vi "engine-step-function.vi"(8 "error in (no error)":errorcluster, 9 "isRunning?":bool=TRUE, 10 "clk":dbl, 11 "HeaderElement in":cluster{variant[]}) -> (0 "error out":errorcluster, 1 "ENG.CALL":cluster{"CMD":T1, "data":variant}={"CMD"=enum."ENG.PROC.ISRUNNING", "data"=variant}, 2 "Next State in":cluster{"CMD":T2, "data":variant}={"CMD"=enum."JUMP", "data"=variant}, 3 "HeaderElement out":cluster{variant[]}, 4 "continue?":bool)   [LabVIEW 2024]
uses:
  controls/typeCmdPostStepFunc.ctl
  controls/state-engine.ctl
  controls/typeProcVarientName.ctl
  controls/type.StepFunction.ctl
  controls/enumVarCtrlIO.ctl
  controls/enum.io.mode.ctl
  controls/enum.io.type.ctl
  controls/IONode.ctl
  controls/type.address.ctl
  controls/typeXyPoint.ctl
  controls/typeStepVarients.ctl
  controls/typePathSelector.ctl
  controls/enum-q-sched.ctl
  controls/cluster-q-sched.ctl
  controls/type.eng.proc.isrunning.ctl
  controls/type.eng-call.proc-insert.ctl
  Polymorphics/variantCtrlStepFunction.vi
  Polymorphics/variantCtrlString.vi
  Polymorphics/variantCtrlSetpoint.vi
  Polymorphics/variantCtrlNumber.vi
  <vilib>/Utility/error.llb/Trim Whitespace.vi
  <vilib>/Utility/error.llb/Trim Whitespace One-Sided.vi
  Polymorphics/enumToStr.ProcHead.vi
  util.error.create.vi
  Polymorphics/variantCtrlStepPath.vi
  globals/globals-engine.vi
  util.environment.vi
  util-address-builder.vi
  util.DO.ToString.vi
  Polymorphics/io.command-builder.vi
  Polymorphics/io.command-builder.DO.vi
  Polymorphics/io.command-builder.AI.vi
  Polymorphics/io.command-builder.DI.vi
  io.frame.vi
  io.visa.vi
  io.responseValidator.vi
  Polymorphics/io.command-parser.DI.vi
  Polymorphics/io.command-parser.AI.vi
  <vilib>/Utility/libraryn.llb/Create Directory Recursive.vi
  Polymorphics/variantCtrlStepPointer.vi
  <vilib>/Utility/file.llb/Write Delimited Spreadsheet (string).vi
  Polymorphics/variantCtrlStepUserMessage.vi
  Polymorphics/variantCtrlStepProcPointer.vi
  Polymorphics/enumToStr.Step.vi
panel:
  out "DI":bool[](array[boolean])
  in  "deltaClk(global def)":dbl
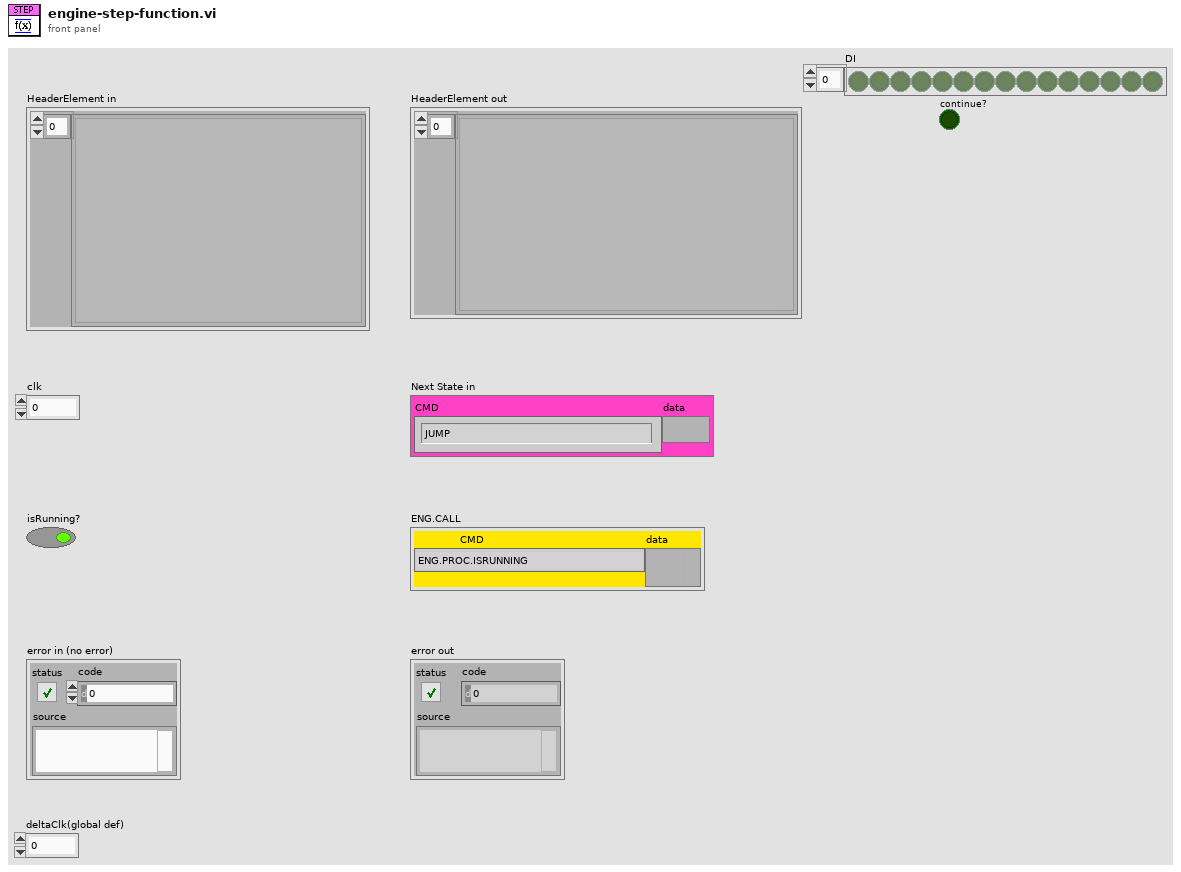
[diagram p1: front panel]
types:
  T1 = typedef "state-engine.ctl" = enum16{"ENG.NO-OP", "ENG.START", "ENG.STOP", "ENG.EXECUTE", "ENG.STATUS", "ENG.EXTERNAL-CALL", "ENG.INIT", "ENG.INIT.VARS", "ENG.INIT.SERIAL", "ENG.LOAD", "ENG.LOAD.SINGLE", "ENG.LOAD.MODULE", "ENG.LOAD.RELOAD", "ENG.LOAD.UNLOAD", "ENG.IO.LOAD", "ENG.IO.SAVE", "ENG.PROC.RELOAD-BY-NAME", "ENG.PROC.START", "ENG.PROC.STOP", "ENG.PROC.INSERT-STEPS", "ENG.PROC.ISRUNNING", "ENG.PROC.PRESET", "ENG.PROC.STATUS", "ENG.PRINT-USER-MSG", "ENG.RIO.SNAPSHOT", "ENG.RIO.AIN-SNAPSHOT-CALIB", "ENG.RIO.DOUT-BY-ADDR", "ENG.RIO.DOUT-BY-NAME", "ENG.RIO.RFS-DELAY-SET-X1", "ENG.RIO.RFS-DELAY-SET-X8", "ENG.RIO.RFS-CYCLES-SET", "ENG.RIO.RFS-CYCLES-GET", "ENG.RIO.RFS-ENABLE", "ENG.EXIT"}
  T2 = typedef "typeCmdPostStepFunc.ctl" = enum16{"NEXT", "PREV", "JUMP", "STAY", "COMPLETE", "ENGCALL.PROC.START", "ENGCALL.PROC.STOP", "ENGCALL.PROC.COMPLETION-CHECK", "ENGCALL.PROC.INIT", "ERROR"}
  T3 = typedef "typeProcVarientName.ctl" = enum16{"procNameID", "procModuleID", "procPath", "procIsRunning", "procIndex", "procModule", "procRegisterNumeric", "procRegisterString", "procReport", "procReportPrev", "procCLK", "procStepPointer", "procType"}
  T4 = typedef "enumVarCtrlIO.ctl" = enum16{"IO Get By Key", "IO List Configs", "IO Add By Key", "IO Modify Value By Key", "IO Modify Calib By Key", "IO Modify ADDR By Key", "IO Modify Mode By Key", "IO Modify Type By Key", "IO Modify Name By Key", "IO Remove By Key", "IO Remove All"}
  T5 = typedef "IONode.ctl" = cluster{"ADDR":T6, "Label":string, "Type":T7, "Mode":T8, "Value":string, "Tags":string, "calibration":T9[]}
  T6 = typedef "type.address.ctl" = u16
  T7 = typedef "enum.io.type.ctl" = enum16{"Type", "DI", "DO", "AI", "AO", "VL", "BUF"}
  T8 = typedef "enum.io.mode.ctl" = enum16{"Mode", "RIO", "SIM"}
  T9 = typedef "typeXyPoint.ctl" = cluster{"X":dbl, "Y":dbl}
  T10 = typedef "typeStepVarients.ctl" = enum16{"stepNameID", "stepFunction", "stepReport", "stepSetpoint", "stepPointer", "stepProcPointer", "stepIoPointer", "stepIoValue", "stepFilePointer", "stepMessage", "stepTimeString", "stepNumReg", "stepStrReg", "stepSeconds", "stepUnitDoseParams", "stepUnitIndex"}
  T11 = typedef "typePathSelector.ctl" = enum16{"DIR_PROCS", "DIR_CONFIG", "DIR_TEMPLATE", "DIR_IO_FILE", "DIR_RECORD", "DIR_LOG", "DIR_RUNTIME", "DIR_PRESET", "DIR_INI"}
  T12 = typedef "cluster-q-sched.ctl" = cluster{"Proc Name":string, "value":cluster{"Enable":bool, "Time":timestamp}}
  T13 = typedef "enum-q-sched.ctl" = enum16{"SCHED.INIT", "SCHED.REGISTER", "SCHED.EXIT"}
  T14 = typedef "type.eng.proc.isrunning.ctl" = cluster{"callerProc":string, "procPointer":string}
  T15 = typedef "type.eng-call.proc-insert.ctl" = cluster{"ProcName":string, "instructions":variant[]}
  T16 = typedef "type.StepFunction.ctl" = enum16{"__NO-OP", "_DELAY_LOAD", "_DELAY_COMPARE", "_JUMP", "_COMPLETE", "_COMPARE", "_LOG_MESSAGE", "_LOG_LAST_REPORT", "_SCHEDULE", "_SCHEDULE_DAILY", "CLK_COMPARE", "PROC_START", "PROC_STOP", "PROC_LOAD", "PROC_COMPLETION_CHECK", "PROC_COMPLETION_LOAD", "_IO_READ", "_IO_READ_MANY", "_IO_WRITE", "_IO_WRITE_BY_REG", "_IO_GET_OUTPUT", "_OCS_CHECK", "_OCS_RECORD", "_GET_RH", "_GET_ACC_UV", "_GET_WD", "_GET_WS", "_REC_DELETE", "_REC_MOVE", "_REC_COPY", "_IRR_CHECK", "UNIT_CHECK", "UNIT_SAMPLE", "UNIT_DOSE"}
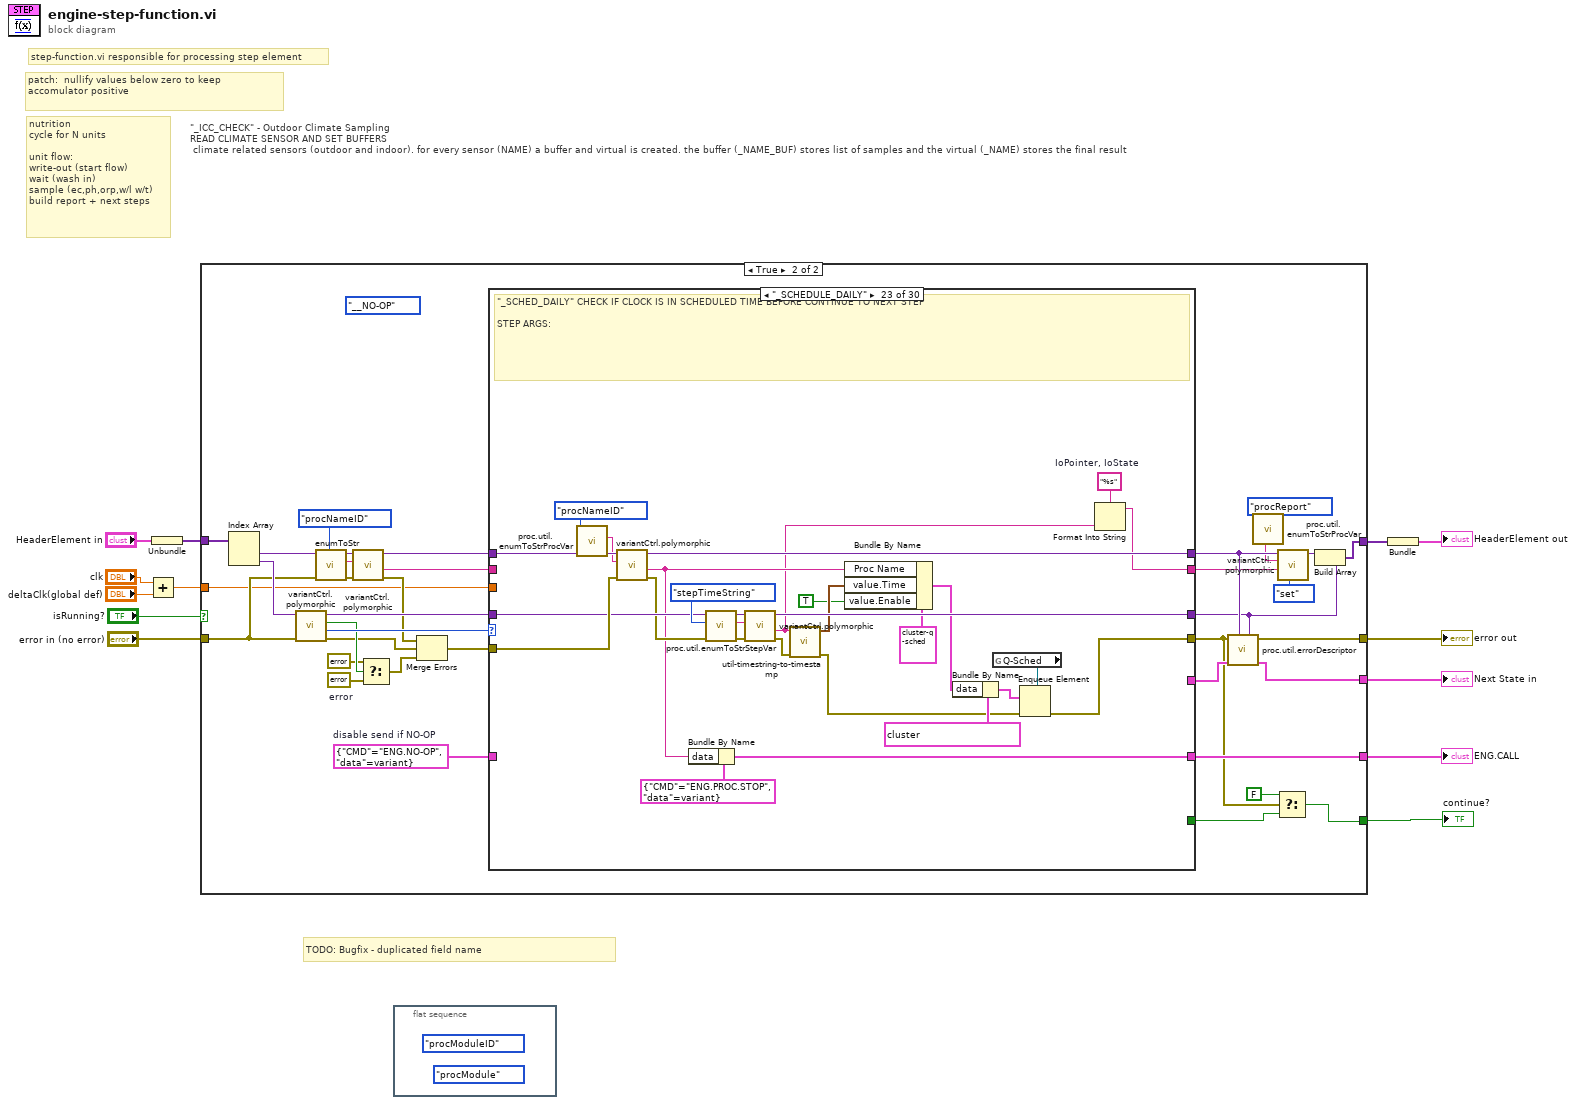
[diagram p0: block diagram]
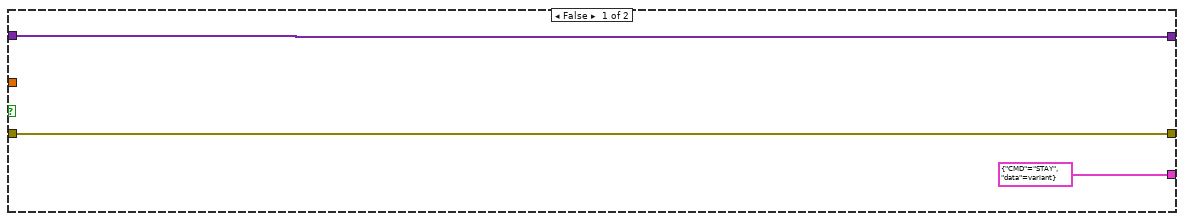
[diagram p2: hidden frame]
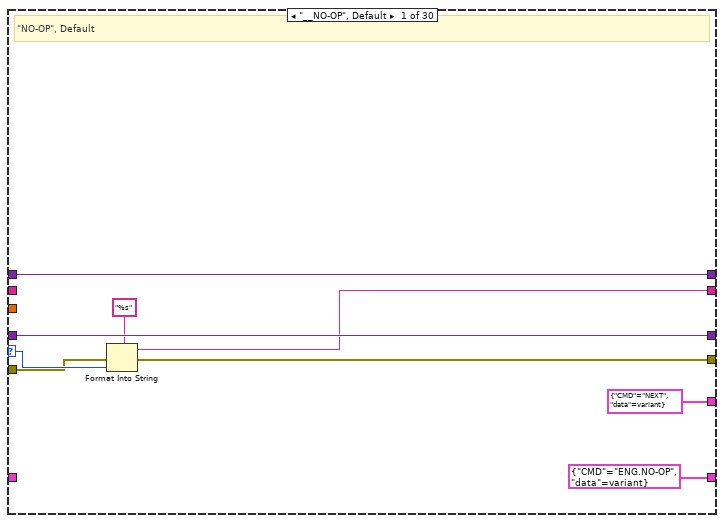
[diagram p3: hidden frame]
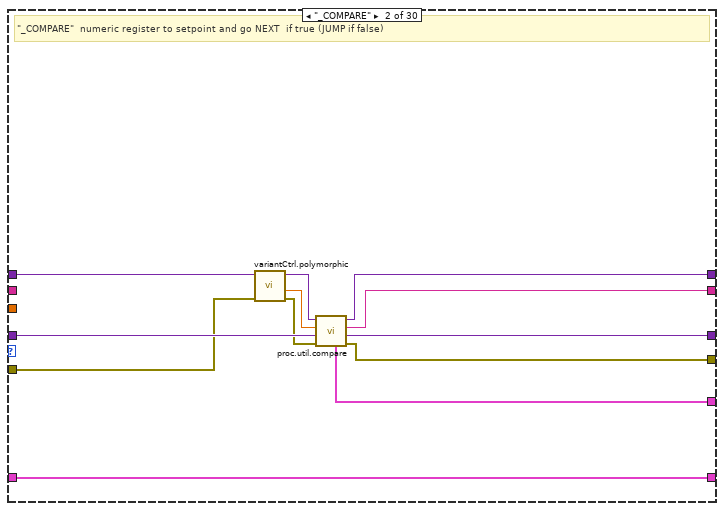
[diagram p4: hidden frame]
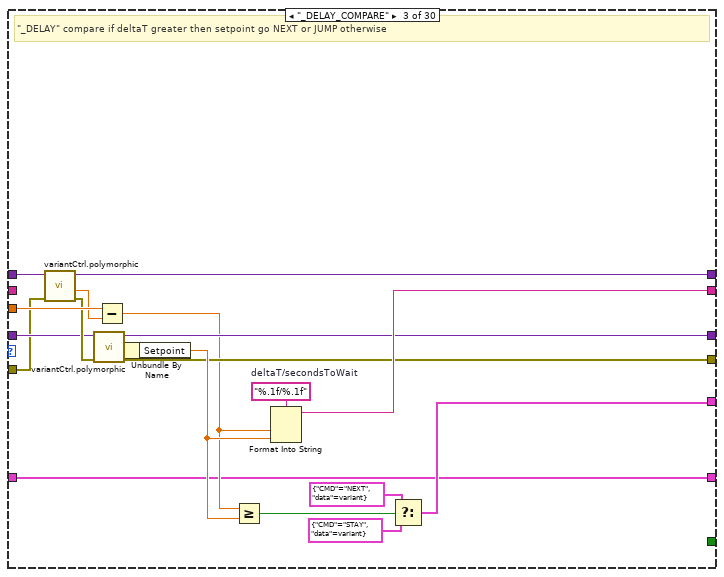
[diagram p5: hidden frame]
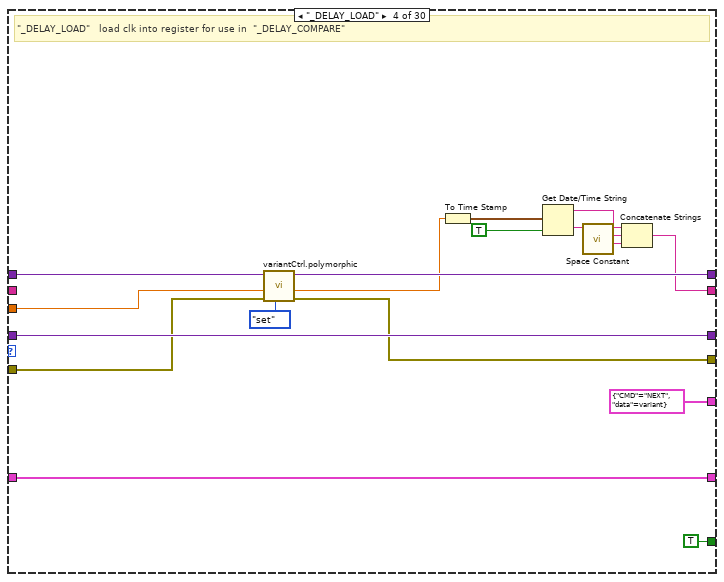
[diagram p6: hidden frame]
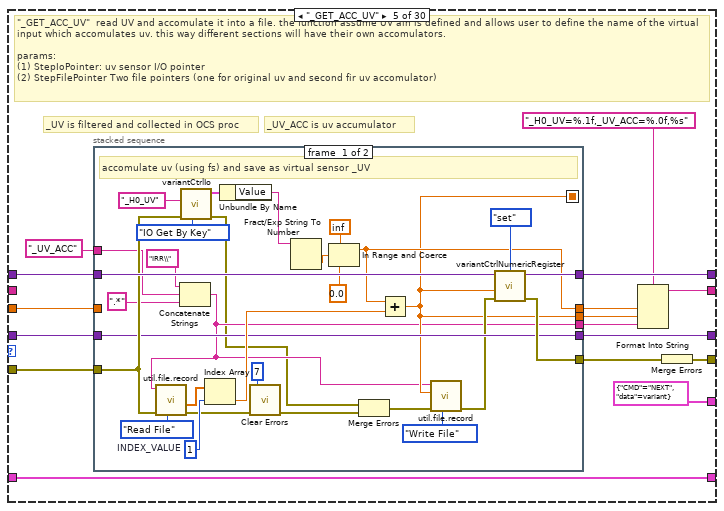
[diagram p7: hidden frame]
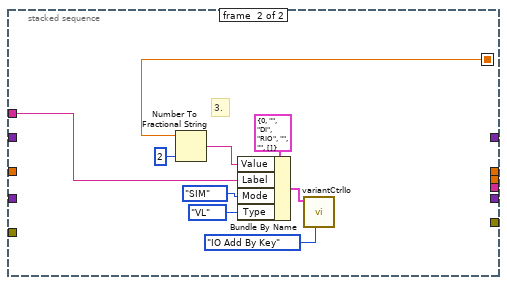
[diagram p8: hidden frame]
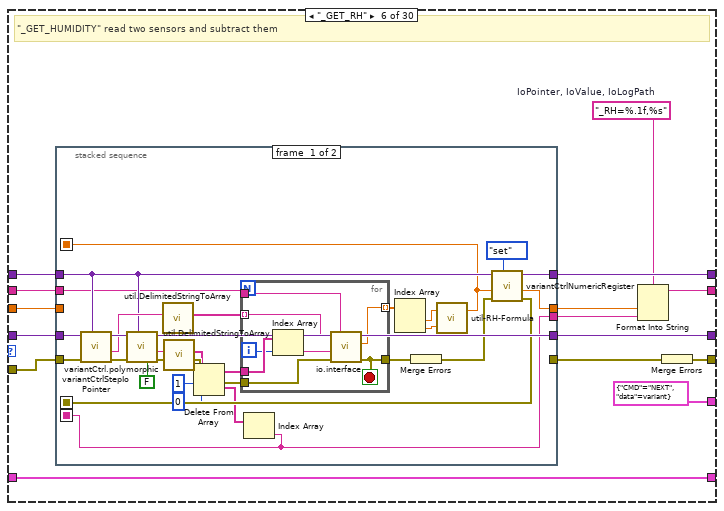
[diagram p9: hidden frame]
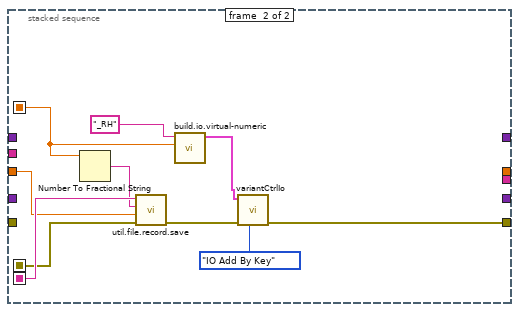
[diagram p10: hidden frame]
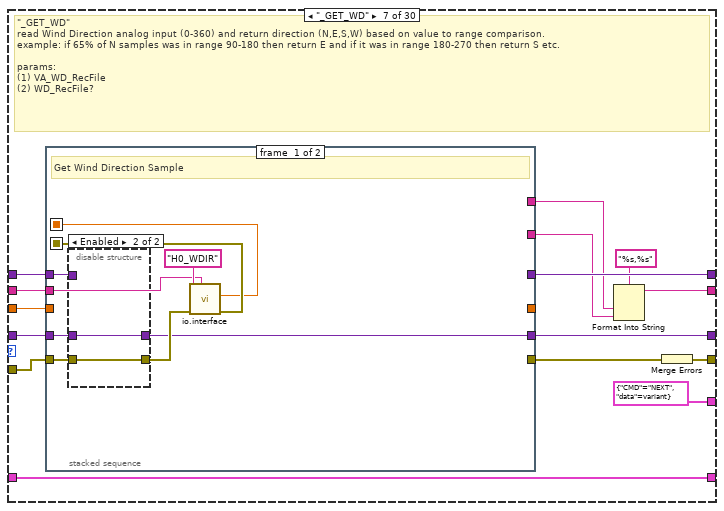
[diagram p11: hidden frame]
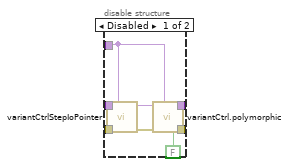
[diagram p12: hidden frame]
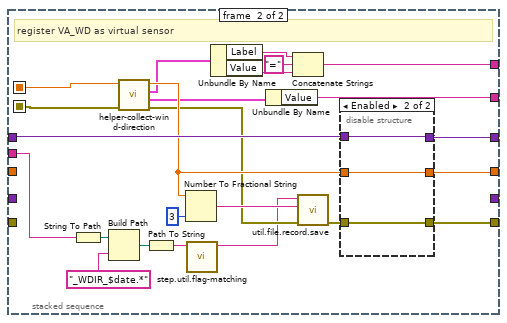
[diagram p13: hidden frame]
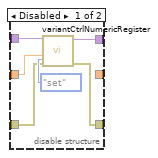
[diagram p14: hidden frame]
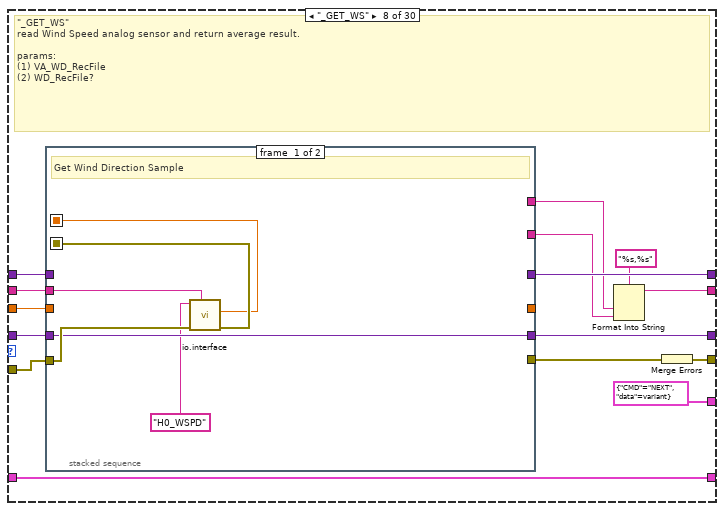
[diagram p15: hidden frame]
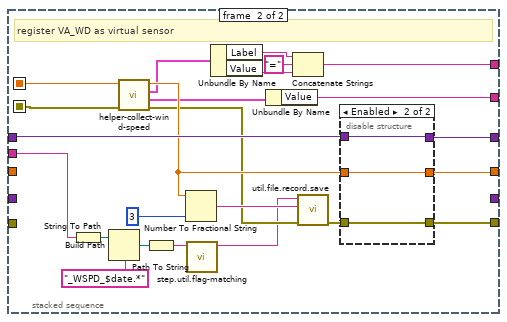
[diagram p16: hidden frame]
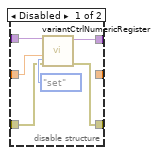
[diagram p17: hidden frame]
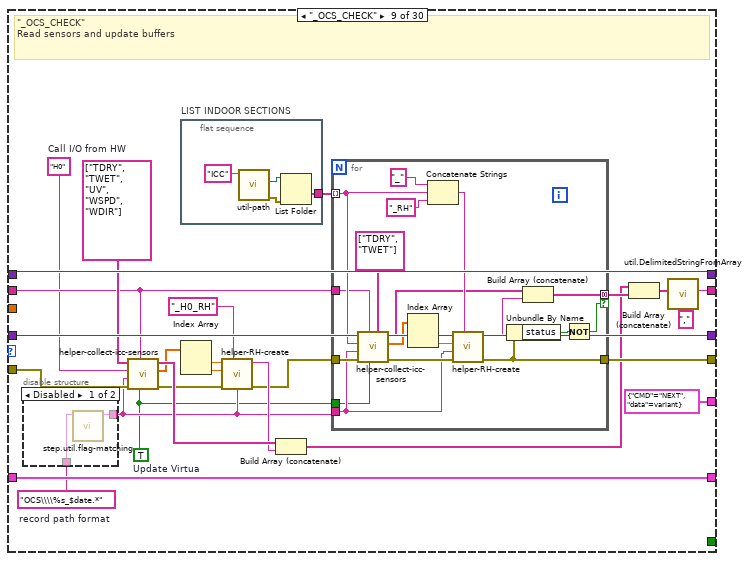
[diagram p18: hidden frame]
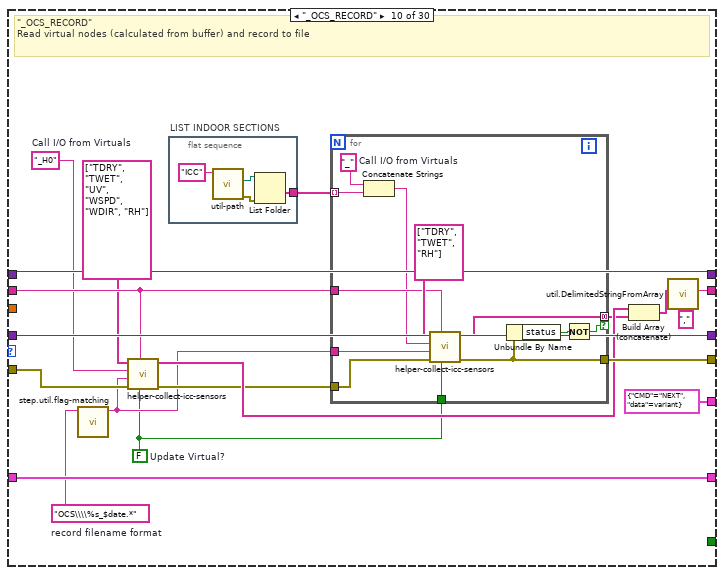
[diagram p20: hidden frame]
diagram:
  # "TODO: Bugfix - duplicated field name"
  # "\"_ICC_CHECK\" - Outdoor Climate Sampling\nREAD CLIMATE SENSOR AND SET BUFFERS\n climate related sensors (outdoor and indoor). for every sensor (NAME) a buffer and virtual is created. the buffer (_NAME_BUF) stores list of samples and the virtual (_NAME) stores the final result"
  # "patch:  nullify values below zero to keep accomulator positive"
  # "nutrition\ncycle for N units\n\nunit flow:\nwrite-out (start flow)\nwait (wash in)\nsample (ec,ph,orp,w/l w/t)\nbuild report + next steps"
  # "step-function.vi responsible for processing step element"
  n1 = Add(x="clk", y="deltaClk(global def)") -> (x+y=w2:dbl)
  n2 = Unbundle("HeaderElement in") -> (w7:variant[])
  n3 = case shown="True" "isRunning?" {
    tunnel: [cluster{"CMD":T2, "data":variant} {"CMD"=enum."STAY", "data"=variant} ("Next State") w33] -> w13
    tunnel: [w15 w32] -> w12
    tunnel: [w16 w46] -> w11
    tunnel: w7 -> [w16 w39]
    tunnel: "error in (no error)" -> [w15 w37]
    tunnel: w2 -> [_ w35]
    tunnel: [_ w27] -> w5
    tunnel: [_ w17] -> w1
    frame False {
    }
    frame True {
      w26 = cluster{"CMD":T1, "data":variant} {"CMD"=enum."ENG.NO-OP", "data"=variant}  # disable send if NO-OP
      (unwired) type.StepFunction."__NO-OP" ("Operation out")
      w44 = errorcluster {"status"=TRUE, "code"=-1, "source"="Missing stepFunction "}  # error
      n4 = Index Array(array=w39) -> (element #1=w40:variant, element #2=w38:variant)  [unwired: 2 in]
      n5 = call-poly "variantCtrl.polymorphic.vi"("error in"=w37, "variant in"=w38) -> ("error out"=w41:errorcluster, "StepFunction"=w50:T16, "found/replaced"=w45:bool, "variant out"=w51:variant)  [unwired: 6 in]
      n6 = call-poly "enumToStr.vi"("Proc var"=typeProcVarientName."procNameID" ("proc var")) -> ("String"=w21:string)  [unwired: 10 in]
      n7 = call-poly "variantCtrl.polymorphic.vi"("error in"=w37, "name in"=w21, "Step in"=w40) -> ("error out"=w36:errorcluster, "String Value"=w24:string, "Step out"=w49:variant)  [unwired: 5 in, 1 out]
      n8 = Select(t=errorcluster {"status"=FALSE, "code"=0, "source"=""}, s=w45, f=w44) -> (s? t:f=w43:errorcluster)
      n9 = Merge Errors(w36, w41, w43) -> (w48:errorcluster)
      n10 = case "Step Functions" shown="\"_SCHEDULE_DAILY\"" w50 {
        selector: w50 -> [w57 _ _ _ _ _ _ _ _ _ _ _ _ _ _ _ _ _ _ _ w728 _ _ _ _ _ w864 _ _ _]
        tunnel: w51 -> [w59 w67 w82 w108 w121 w175 w236 w303 w370 w414 w446 w493 w524 w554 w576 w587 w613 w621 w650 w663 w746 w769 w787 w802 w826 w860 w870 w892 w911 w968]
        tunnel: [w53 w66 w80 w105 w116 w170 w231 w298 w363 w410 w442 w489 w519 w549 w574 w580 w608 w616 w644 w661 w741 w768 w785 w800 w817 w838 w868 w881 w906 w958] -> w20
        tunnel: [w59 w69 w81 w108 w122 w176 w237 w304 w370 w414 w447 w494 w523 w551 w575 w588 w612 w621 w651 w658 w747 w771 w788 w805 w825 w859 w869 w893 w912 w969] -> w30
        tunnel: w35 -> [_ _ w91 w100 w114 w168 w229 w296 _ _ _ _ _ _ _ w594 _ _ _ _ _ w764 _ w803 _ _ _ w879 _ _]
        tunnel: w49 -> [w60 w71 w87 w107 w120 w174 w235 w302 w369 w413 w444 w491 w522 w545 w568 w595 w611 w618 w649 w659 w745 w763 w794 w806 w821 w853 w862 w896 w914 w972]
        tunnel: [w60 w72 w83 w106 w123 w177 w238 w305 w369 w413 w448 w495 w522 w545 w569 w595 w611 w619 w654 w665 w745 w763 w795 w807 w822 w840 w862 w896 w914 w972] -> w31
        tunnel: [w55 w64 w88 w94 w117 w171 w232 w299 w366 w411 w450 w498 w512 w558 w577 w593 w606 "completed" ("status") w639 w660 w742 w767 w774 w799 w813 w851 w861 w884 w904 w957] -> w22
        tunnel: [cluster{"CMD":T2, "data":variant} {"CMD"=enum."NEXT", "data"=variant} ("Next State") w68 w77 cluster{"CMD":T2, "data":variant} {"CMD"=enum."NEXT", "data"=variant} ("Next State") cluster{"CMD":T2, "data":variant} {"CMD"=enum."NEXT", "data"=variant} ("Next State") cluster{"CMD":T2, "data":variant} {"CMD"=enum."NEXT", "data"=variant} ("Next State") cluster{"CMD":T2, "data":variant} {"CMD"=enum."NEXT", "data"=variant} ("Next State") cluster{"CMD":T2, "data":variant} {"CMD"=enum."NEXT", "data"=variant} ("Next State") cluster{"CMD":T2, "data":variant} {"CMD"=enum."NEXT", "data"=variant} ("Next State") cluster{"CMD":T2, "data":variant} {"CMD"=enum."NEXT", "data"=variant} ("Next State") cluster{"CMD":T2, "data":variant} {"CMD"=enum."NEXT", "data"=variant} ("Next State") cluster{"CMD":T2, "data":variant} {"CMD"=enum."NEXT", "data"=variant} ("Next State") cluster{"CMD":T2, "data":variant} {"CMD"=enum."NEXT", "data"=variant} ("Next State") cluster{"CMD":T2, "data":variant} {"CMD"=enum."NEXT", "data"=variant} ("Next State") cluster{"CMD":T2, "data":variant} {"CMD"=enum."NEXT", "data"=variant} ("Next State") w583 w609 cluster{"CMD":T2, "data":variant} {"CMD"=enum."COMPLETE", "data"=variant} ("JUMP") cluster{"CMD":T2, "data":variant} {"CMD"=enum."NEXT", "data"=variant} ("JUMP") w664 cluster{"CMD":T2, "data":variant} {"CMD"=enum."NEXT", "data"=variant} ("Next State") w770 _ w804 w819 cluster{"CMD":T2, "data":variant} {"CMD"=enum."NEXT", "data"=variant} ("Next State") cluster{"CMD":T2, "data":variant} {"CMD"=enum."NEXT", "data"=variant} ("Next State") cluster{"CMD":T2, "data":variant} {"CMD"=enum."NEXT", "data"=variant} ("Next State") w913 cluster{"CMD":T2, "data":variant} {"CMD"=enum."NEXT", "data"=variant} ("Next State")] -> w34
        tunnel: w48 -> [w54 w62 w75 w102 w119 w173 w234 w301 w355 w409 w441 w487 w521 w543 w572 w582 w605 w617 w648 w662 w744 w766 w791 w801 w815 w850 w867 w882 _ _]
        tunnel: [cluster{"CMD":T1, "data":variant} {"CMD"=enum."ENG.NO-OP", "data"=variant} ("element") w61 w73 w101 w110 w165 w228 w295 w368 w412 w440 w484 w520 w541 w570 w591 w604 w620 w628 w657 w726 w765 w796 w798 w809 w848 w865 w889 w909 w963] -> w27
        tunnel: w26 -> [_ w61 w73 w101 w110 w165 w228 w295 w368 w412 w440 w484 w520 w541 w570 w590 w604 w620 w628 w657 w726 w765 _ w798 w809 _ _ w891 w910 w965]
        tunnel: w24 -> [_ _ _ _ _ w164 w227 w294 w351 w408 w432 w480 w510 w538 w561 w589 _ _ _ _ _ _ _ _ _ _ _ w887 w908 w956]
        tunnel: [_ _ _ TRUE _ _ _ _ _ _ _ _ _ TRUE _ _ _ _ _ _ _ _ _ _ _ _ _ _ _ _] -> w18
        frame "__NO-OP", Default {
          # "\"NO-OP\", Default"
          n11 = Format Into String(format string="%s", error in=w54, w57) -> (resulting string=w55:string, error out=w53:errorcluster)  [unwired: 1 in]
        }
        frame "_COMPARE" {
          # "\"_COMPARE\"  numeric register to setpoint and go NEXT  if true (JUMP if false)"
          n12 = call-poly "variantCtrl.polymorphic.vi"("error in"=w62, "procElement"=w71) -> ("error out"=w63:errorcluster, "procNumericRegister out"=w65:dbl, "procElement out"=w70:variant)  [unwired: 7 in]
          n13 = call "proc.util.compare.vi"("error in"=w63, "stepElement in"=w67, "Input"=w65, "procElement in"=w70) -> ("error out"=w66:errorcluster, "stepElement out"=w69:variant, "resulting string"=w64:string, "procElement out"=w72:variant, "Next State"=w68:cluster{"CMD":T2, "data":variant})  [unwired: 3 in]
        }
        frame "_DELAY_COMPARE" {
          w90 = "%.1f/%.1f"  # deltaT/secondsToWait
          # "\"_DELAY\" compare if deltaT greater then setpoint go NEXT or JUMP otherwise"
          n14 = call-poly "variantCtrl.polymorphic.vi"("error in"=w75, "procElement"=w87) -> ("error out"=w86:errorcluster, "procNumericRegister out"=w85:dbl, "procElement out"=w83:variant)  [unwired: 7 in]
          n15 = call-poly "variantCtrl.polymorphic.vi"("error in"=w86, "procElement in in"=w82) -> ("error out"=w80:errorcluster, "setpoint"=w89:cluster{"Comparison":string, "Setpoint":dbl}, "procElement out"=w81:variant)  [unwired: 6 in, 1 out]
          n16 = Subtract(x=w91, y=w85) -> (x-y=w79:dbl)
          n17 = Unbundle By Name(w89) -> ("Setpoint"=w84:dbl)
          n18 = Greater Or Equal?(x=w79, y=w84) -> (x >= y?=w78:bool)
          n19 = Format Into String(format string=w90, w79, w84) -> (resulting string=w88:string)  [unwired: 2 in, 1 out]
          n20 = Select(t=cluster{"CMD":T2, "data":variant} {"CMD"=enum."NEXT", "data"=variant} ("NEXT"), s=w78, f=cluster{"CMD":T2, "data":variant} {"CMD"=enum."STAY", "data"=variant} ("JUMP")) -> (s? t:f=w77:cluster{"CMD":T2, "data":variant})
        }
        frame "_DELAY_LOAD" {
          # "\"_DELAY_LOAD\"   load clk into register for use in  \"_DELAY_COMPARE\""
          n21 = call-poly "variantCtrl.polymorphic.vi"("menu"=enum16{"get", "set"}."set", "error in"=w102, "procNumericRegister in"=w100, "procElement"=w107) -> ("error out"=w105:errorcluster, "procNumericRegister out"=w99:dbl, "procElement out"=w106:variant)  [unwired: 5 in]
          n22 = To Time Stamp(1:w99) -> (0:w98:timestamp)
          n23 = Get Date/Time String(seconds (now)=w98, want seconds? (F)=TRUE) -> (date string=w95:string, time string=w97:string)  [unwired: 1 in]
          n24 = call <vilib>:"Space Constant.vi"() -> ("String"=w96:string)
          n25 = Concatenate Strings(w97, w96, w95) -> (w94:string)
        }
        frame "_GET_ACC_UV" {
          # "_UV_ACC is uv accumulator"
          # "_UV is filtered and collected in OCS proc"
          # "\"_GET_ACC_UV\"  read UV and accomulate it into a file. the function assume UV ain is defined and allows user to define the name of the virtual input which accomulates uv. this way different sections will have their own accomulators. \n\nparams:\n(1) StepIoPointer: uv sensor I/O pointer\n(2) StepFilePointer Two file pointers (one for original uv and second fir uv accomulator)"
          n26 = stacked-sequence {
            seq-local: [w130 _] -> [_ w158]
            tunnel: [w154 _] -> w123
            tunnel: [w137 _] -> w122
            tunnel: w121 -> [w137 _]
            tunnel: w120 -> [w152 _]
            tunnel: w119 -> [w138 _]
            tunnel: [w153 _] -> w115
            tunnel: w114 -> [_ _]
            tunnel: [w132 _] -> w113
            tunnel: [w127 _] -> w112
            tunnel: [w130 _] -> w111
            tunnel: "_UV_ACC" ("Label") -> [w129 w155]
            frame #0 {
              w149 = 1  # INDEX_VALUE
              # "accomulate uv (using fs) and save as virtual sensor _UV"
              n27 = Concatenate Strings("IRR\\" ("string"), w129, ".*" ("$string in")) -> (w127:string)
              n28 = call "util.file.record.vi"("Operation(Read)"=enum16{"Read File", "Write File"}."Read File", "error in"=w138, "path.* in"=w127) -> ("error out"=w147:errorcluster, "Last Record out"=w150:dbl[])  [unwired: 5 in, 2 out]
              n29 = call "variantCtrlIo.vi"("menu (Get Param)"=enumVarCtrlIO."IO Get By Key", "error in"=w138, "Key (use IOnode Label if empty )"="_H0_UV" ("Label")) -> ("error out"=w126:errorcluster, "IOnode out"=w140:T5)  [unwired: 4 in, 3 out]
              n30 = Index Array(array=w150, index=w149) -> (element=w148:dbl)
              n31 = Unbundle By Name(w140) -> ("Value"=w139:string)
              n32 = call <vilib>:"Clear Errors.vi"("error in (no error)"=w147, "specific error code to clear (0: all)"=7) -> ("error out"=w145:errorcluster)  [unwired: 4 in, 1 out]
              n33 = Fract/Exp String To Number(string=w139) -> (number=w135:dbl)  [unwired: 3 in, 1 out]
              n34 = In Range and Coerce(upper limit=inf, x=w135, lower limit=0.0) -> (coerced(x)=w132:dbl)  [unwired: 1 out]
              n35 = Merge Errors(w126, w145) -> (w136:errorcluster)
              n36 = Add(x=w132, y=w148) -> (x+y=w130:dbl)
              n37 = call "util.file.record.vi"("Operation(Read)"=enum16{"Read File", "Write File"}."Write File", "error in"=w136, "value"=w130, "path.* in"=w127) -> ("error out"=w131:errorcluster)  [unwired: 4 in, 3 out]
              n38 = call "variantCtrlNumericRegister.vi"("menu"=enum16{"get", "set"}."set", "error in"=w131, "procNumericRegister in"=w130, "procElement"=w152) -> ("error out"=w153:errorcluster, "procElement out"=w154:variant)  [unwired: 5 in, 1 out]
            }
            frame #1 {
              # "3."
              n39 = Number To Fractional String(number=w158, precision (6)=i16 2) -> (F-format string=w157:string)  [unwired: 2 in]
              n40 = Bundle By Name(cluster=T5 {"ADDR"=0, "Label"="", "Type"=enum."DI", "Mode"=enum."RIO", "Value"="", "Tags"="", "calibration"=[]} ("IoConf in"), "Value"=w157, "Label"=w155, "Mode"=enum.io.mode."SIM", "Type"=enum.io.type."VL" ("type")) -> (w161:T5)
              n41 = call "variantCtrlIo.vi"("menu (Get Param)"=enumVarCtrlIO."IO Add By Key" ("menu in (get)"), "IOnode in"=w161) -> ()  [unwired: 5 in, 5 out]
            }
          }
          n42 = Format Into String(format string="_H0_UV=%.1f,_UV_ACC=%.0f,%s", w113, w111, w112) -> (resulting string=w117:string)  [unwired: 2 in, 1 out]
          n43 = Merge Errors(w115) -> (w116:errorcluster)
        }
        frame "_GET_RH" {
          w172 = "_RH=%.1f,%s"  # IoPointer, IoValue, IoLogPath
          # "\"_GET_HUMIDITY\" read two sensors and subtract them"
          n44 = stacked-sequence {
            seq-local: [w180 _] -> [_ w216]
            seq-local: [w190 _] -> [_ w221]
            seq-local: [w186 _] -> [_ w222]
            tunnel: [w195 _] -> w177
            tunnel: [w194 _] -> w176
            tunnel: w175 -> [w204 _]
            tunnel: w174 -> [w193 _]
            tunnel: w173 -> [w202 _]
            tunnel: [_ w224] -> w169
            tunnel: w168 -> [_ w220]
            tunnel: [w189 _] -> w167
            tunnel: [w186 _] -> w166
            tunnel: w164 -> [w179 _]
            frame #0 {
              n45 = call "variantCtrlStepIoPointer.vi"("procElement"=w193, "error in"=w202, "StepElement in"=w204) -> ("error out"=w205:errorcluster, "I/O Pointer out"=w198:string, "stepElement out"=w203:variant)  [unwired: 5 in, 1 out]
              n46 = call-poly "variantCtrl.polymorphic.vi"("isRequired (T)"=FALSE, "procElement"=w193, "error in (no error)"=w205, "stepElement in"=w203) -> ("error out"=w206:errorcluster, "File Pointer out"=w196:string, "step\\element out"=w194:variant)  [unwired: 5 in]
              n47 = call "util.DelimitedStringToArray.vi"("delimitaed string"=w198) -> ("array out"=w197:string[])  [unwired: 10 in]
              n48 = call "util.DelimitedStringToArray.vi"("delimitaed string"=w196) -> ("array out"=w192:string[])  [unwired: 10 in]
              n49 = Delete From Array(array=w192, length=1, index=0) -> (deleted portion=w185:string[], array with subset deleted=w184:string[])
              n50 = for {
                tunnel: [w212] -> w199 mode=indexing
                tunnel: w197 -> [w213] mode=indexing
                tunnel: w184 -> [w210]
                tunnel: w206 -> [w214]
                tunnel: [w211] -> w200
                tunnel: w179 -> [w207]
                i -> [w209]
                stop <- w211 stop-if-true
                n51 = Index Array(array=w210, index=w209) -> (element=w208:string)
                n52 = call "io.interface.vi"("Caller"=w207, "error in"=w214, "record filename.* (disabled if empty)"=w208, "IO Name in"=w213) -> ("error out"=w211:errorcluster, "Value out"=w212:dbl)  [unwired: 2 in, 4 out]
              }
              n53 = Index Array(array=w185) -> (element=w186:string)  [unwired: 1 in]
              n54 = Index Array(array=w199) -> (element #1=w182:dbl, element #2=w181:dbl)  [unwired: 2 in]
              n55 = Merge Errors(w200) -> (w191:errorcluster)
              n56 = call "util-RH-Formula.vi"("Twet"=w181, "Tdry"=w182) -> ("RH"=w180:dbl)  [unwired: 1 out]
              n57 = call "variantCtrlNumericRegister.vi"("menu"=enum16{"get", "set"}."set", "error in"=w191, "procNumericRegister in"=w180, "procElement"=w193) -> ("error out"=w190:errorcluster, "procNumericRegister out"=w189:dbl, "procElement out"=w195:variant)  [unwired: 5 in]
            }
            frame #1 {
              n58 = Number To Fractional String(number=w216) -> (F-format string=w219:string)  [unwired: 3 in]
              n59 = call "util.file.record.save.vi"("error in"=w221, "clk(NaN)"=w220, "String Delimited Values"=w219, "record path in"=w222) -> ("error out"=w218:errorcluster)  [unwired: 6 in, 1 out]
              n60 = call "build.io.virtual-numeric.vi"("Numeric Value"=w216, "Label"="_RH" ("Virtual _RH")) -> ("IoConf out"=w215:T5)  [unwired: 9 in]
              n61 = call "variantCtrlIo.vi"("menu (Get Param)"=enumVarCtrlIO."IO Add By Key" ("menu in (get)"), "error in"=w218, "IOnode in"=w215) -> ("error out"=w224:errorcluster)  [unwired: 4 in, 4 out]
            }
          }
          n62 = Format Into String(format string=w172, w167, w166) -> (resulting string=w171:string)  [unwired: 2 in, 1 out]
          n63 = Merge Errors(w169) -> (w170:errorcluster)
        }
        frame "_GET_WD" {
          # "\"_GET_WD\" \nread Wind Direction analog input (0-360) and return direction (N,E,S,W) based on value to range comparison. \nexample: if 65% of N samples was in range 90-180 then return E and if it was in range 180-270 then return S etc. \n\nparams:\n(1) VA_WD_RecFile\n(2) WD_RecFile?"
          n64 = stacked-sequence {
            seq-local: [w242 _] -> [_ w279]
            seq-local: [w243 _] -> [_ w266]
            tunnel: [_ w282] -> w238
            tunnel: [w245 _] -> w237
            tunnel: w236 -> [w247 _]
            tunnel: w235 -> [w244 w280]
            tunnel: w234 -> [w246 _]
            tunnel: [_ w281] -> w230
            tunnel: w229 -> [_ _]
            tunnel: [_ w278] -> _
            tunnel: w227 -> [w240 w272]
            tunnel: [_ w264] -> w225
            tunnel: [_ w259] -> w226
            frame #0 {
              # "Get Wind Direction Sample"
              n65 = disable-structure shown="Enabled" {
                disable-tunnel: [w256 w257] -> w248
                disable-tunnel: w247 -> [w254 w258]
                disable-tunnel: w246 -> [w252 w257]
                disable-tunnel: [w250 w258] -> w245
                disable-tunnel: w244 -> [w249 _]
                frame Disabled {
                  n66 = call "variantCtrlStepIoPointer.vi"("procElement"=w249, "error in"=w252, "StepElement in"=w254) -> ("error out"=w255:errorcluster, "stepElement out"=w253:variant)  [unwired: 5 in, 2 out]
                  n67 = call-poly "variantCtrl.polymorphic.vi"("isRequired (T)"=FALSE, "procElement"=w249, "error in (no error)"=w255, "stepElement in"=w253) -> ("error out"=w256:errorcluster, "step\\element out"=w250:variant)  [unwired: 5 in, 1 out]
                }
                frame Enabled {
                }
              }
              n68 = call "io.interface.vi"("Caller"=w240, "error in"=w248, "IO Name in"="H0_WDIR") -> ("error out"=w243:errorcluster, "Value out"=w242:dbl)  [unwired: 3 in, 4 out]
            }
            frame #1 {
              # "register VA_WD as virtual sensor"
              n69 = String To Path(string=w272) -> (path=w271:path)
              n70 = Build Path(base path=w271, name or relative path="_WDIR_$date.*" ("record path in")) -> (appended path=w269:path)
              n71 = call "helper-collect-wind-direction.vi"("error in"=w266, "Value in"=w279) -> ("error out"=w274:errorcluster, "BUF Node"=w265:T5, "Result Node"=w263:T5, "Result"=w276:dbl)  [unwired: 6 in]
              n72 = Path To String(path=w269) -> (string=w268:string)
              n73 = Number To Fractional String(number=w276, precision (6)=i16 3) -> (F-format string=w275:string)  [unwired: 2 in]
              n74 = call "step.util.flag-matching.vi"("$string in"=w268) -> ("formated string out"=w267:string)  [unwired: 10 in]
              n75 = Unbundle By Name(w263) -> ("Label"=w262:string, "Value"=w261:string)
              n76 = Unbundle By Name(w265) -> ("Value"=w264:string)
              n77 = Concatenate Strings(w262, "=" ("string"), w261) -> (w259:string)
              n78 = call "util.file.record.save.vi"("error in"=w274, "String Delimited Values"=w275, "record path in"=w267) -> ("error out"=w273:errorcluster)  [unwired: 7 in, 1 out]
              n79 = disable-structure shown="Enabled" {
                disable-tunnel: [w288 w291] -> w282
                disable-tunnel: [w287 w290] -> w281
                disable-tunnel: w280 -> [w285 w291]
                disable-tunnel: w276 -> [w284 w289]
                disable-tunnel: w273 -> [w283 w290]
                disable-tunnel: [_ w289] -> w278
                frame Disabled {
                  n80 = call "variantCtrlNumericRegister.vi"("menu"=enum16{"get", "set"}."set", "error in"=w283, "procNumericRegister in"=w284, "procElement"=w285) -> ("error out"=w287:errorcluster, "procElement out"=w288:variant)  [unwired: 5 in, 1 out]
                }
                frame Enabled {
                }
              }
            }
          }
          n81 = Format Into String(format string="%s,%s", w226, w225) -> (resulting string=w232:string)  [unwired: 2 in, 1 out]
          n82 = Merge Errors(w230) -> (w231:errorcluster)
        }
        frame "_GET_WS" {
          # "\"_GET_WS\" \nread Wind Speed analog sensor and return average result. \n\nparams:\n(1) VA_WD_RecFile\n(2) WD_RecFile?"
          n83 = stacked-sequence {
            seq-local: [w309 _] -> [_ w333]
            seq-local: [w310 _] -> [_ w320]
            tunnel: [_ w336] -> w305
            tunnel: [w311 _] -> w304
            tunnel: w303 -> [w311 _]
            tunnel: w302 -> [_ w334]
            tunnel: w301 -> [w312 _]
            tunnel: [_ w335] -> w297
            tunnel: w296 -> [_ _]
            tunnel: [_ w332] -> _
            tunnel: w294 -> [w307 w326]
            tunnel: [_ w318] -> w292
            tunnel: [_ w313] -> w293
            frame #0 {
              # "Get Wind Direction Sample"
              n84 = call "io.interface.vi"("Caller"=w307, "error in"=w312, "IO Name in"="H0_WSPD") -> ("error out"=w310:errorcluster, "Value out"=w309:dbl)  [unwired: 3 in, 4 out]
            }
            frame #1 {
              # "register VA_WD as virtual sensor"
              n85 = String To Path(string=w326) -> (path=w325:path)
              n86 = Build Path(base path=w325, name or relative path="_WSPD_$date.*" ("record path in")) -> (appended path=w323:path)
              n87 = call "helper-collect-wind-speed.vi"("error in"=w320, "Value in"=w333) -> ("error out"=w328:errorcluster, "_W_DIR_BUF Node"=w319:T5, "_W_DIR Node"=w317:T5, "Result"=w330:dbl)  [unwired: 6 in]
              n88 = Path To String(path=w323) -> (string=w322:string)
              n89 = Number To Fractional String(number=w330, precision (6)=i16 3) -> (F-format string=w329:string)  [unwired: 2 in]
              n90 = call "step.util.flag-matching.vi"("$string in"=w322) -> ("formated string out"=w321:string)  [unwired: 10 in]
              n91 = Unbundle By Name(w317) -> ("Label"=w316:string, "Value"=w315:string)
              n92 = Unbundle By Name(w319) -> ("Value"=w318:string)
              n93 = Concatenate Strings(w316, "=" ("string"), w315) -> (w313:string)
              n94 = call "util.file.record.save.vi"("error in"=w328, "String Delimited Values"=w329, "record path in"=w321) -> ("error out"=w327:errorcluster)  [unwired: 7 in, 1 out]
              n95 = disable-structure shown="Enabled" {
                disable-tunnel: [w342 w345] -> w336
                disable-tunnel: [w341 w344] -> w335
                disable-tunnel: w334 -> [w339 w345]
                disable-tunnel: w330 -> [w338 w343]
                disable-tunnel: w327 -> [w337 w344]
                disable-tunnel: [_ w343] -> w332
                frame Disabled {
                  n96 = call "variantCtrlNumericRegister.vi"("menu"=enum16{"get", "set"}."set", "error in"=w337, "procNumericRegister in"=w338, "procElement"=w339) -> ("error out"=w341:errorcluster, "procElement out"=w342:variant)  [unwired: 5 in, 1 out]
                }
                frame Enabled {
                }
              }
            }
          }
          n97 = Format Into String(format string="%s,%s", w293, w292) -> (resulting string=w299:string)  [unwired: 2 in, 1 out]
          n98 = Merge Errors(w297) -> (w298:errorcluster)
        }
        frame "_OCS_CHECK" {
          w346 = TRUE  # Update Virtua
          w347 = "OCS\\\\%s_$date.*"  # record path format
          w350 = "H0"  # Call I/O from HW
          # "\"_OCS_CHECK\" \nRead sensors and update buffers"
          n99 = disable-structure shown="Disabled" {
            disable-tunnel: [w373 _] -> w352
            disable-tunnel: w347 -> [w372 _]
            frame Disabled {
              n100 = call "step.util.flag-matching.vi"("$string in"=w372) -> ("formated string out"=w373:string)  [unwired: 10 in]
            }
            frame Enabled {
            }
          }
          n101 = call "helper-collect-icc-sensors.vi"("Update Virtual? (T)"=w346, "Caller"=w351, "error in"=w355, "path format (ie. OCS\\\\DB\\\\%s.*)"=w352, "Section (IOnode prefix)"=w350, "IOnodes (AI)"=string[] ["TDRY", "TWET", "UV", "WSPD", "WDIR"]) -> ("error out"=w359:errorcluster, "results numeric"=w362:dbl[], "results report"=w365:string[])  [unwired: 3 in]
          n102 = flat-sequence "LIST INDOOR SECTIONS" {
            tunnel: [w374] -> w358
            frame #0 {
              n103 = call "util-path.vi"("append path (ie. folder\\filename.*)"="ICC" ("dir name")) -> ("error out"=w375:errorcluster, "SelectedPath"=w376:path)  [unwired: 6 in, 3 out]
              n104 = List Folder(path=w376, error in=w375) -> (folder names=w374:string[])  [unwired: 2 in, 3 out]
            }
          }
          n105 = Index Array(array=w362) -> (element #1=w361:dbl, element #2=w360:dbl)  [unwired: 2 in]
          n106 = call "helper-RH-create.vi"("Virtual Name"="_H0_RH", "error in"=w359, "record path format OCS\\DB\\%s.* (DISABLE IF EMPTY)"=w352, "Twet"=w360, "Tdry"=w361) -> ("error out"=w348:errorcluster, "result"=w353:string)  [unwired: 4 in, 1 out]
          n107 = Build Array (concatenate)(w365, w353) -> (w354:string[])
          n108 = for {
            tunnel: w358 -> [w391] mode=indexing
            tunnel: w348 -> [w396]
            tunnel: [w383] -> w363
            tunnel: [w386] -> w356 mode=concatenating if=w381
            tunnel: w352 -> [w380]
            tunnel: w351 -> [w379]
            tunnel: w346 -> [w378]
            n109 = call "helper-collect-icc-sensors.vi"("Update Virtual? (T)"=w378, "Caller"=w379, "error in"=w396, "path format (ie. OCS\\\\DB\\\\%s.*)"=w380, "Section (IOnode prefix)"=w391, "IOnodes (AI)"=string[] ["TDRY", "TWET"]) -> ("error out"=w389:errorcluster, "results numeric"=w392:dbl[], "results report"=w387:string[])  [unwired: 3 in]
            n110 = Index Array(array=w392) -> (element #1=w393:dbl, element #2=w394:dbl)  [unwired: 2 in]
            n111 = Concatenate Strings("_" ("string"), w391, "_RH" ("string")) -> (w388:string)
            n112 = call "helper-RH-create.vi"("Virtual Name"=w388, "error in"=w389, "record path format OCS\\DB\\%s.* (DISABLE IF EMPTY)"=w380, "Twet"=w394, "Tdry"=w393) -> ("error out"=w383:errorcluster, "result"=w385:string)  [unwired: 4 in, 1 out]
            n113 = Unbundle By Name(w383) -> ("status"=w382:bool)
            n114 = Build Array (concatenate)(w387, w385) -> (w386:string[])
            n115 = Not(x=w382) -> (.not. x?=w381:bool)
          }
          n116 = Build Array (concatenate)(w354, w356) -> (w357:string[])
          n117 = call "util.DelimitedStringFromArray.vi"("delimiter (Comma)"="," ("delimiter (Tab)"), "params array in"=w357) -> ("delimited string out"=w366:string)  [unwired: 9 in]
        }
        frame "_OCS_RECORD" {
          w398 = "_H0"  # Call I/O from Virtuals
          w397 = FALSE  # Update Virtual?
          w400 = "OCS\\\\%s_$date.*"  # record filename format
          # "\"_OCS_RECORD\"\nRead virtual nodes (calculated from buffer) and record to file"
          n118 = call "step.util.flag-matching.vi"("$string in"=w400) -> ("formated string out"=w399:string)  [unwired: 10 in]
          n119 = call "helper-collect-icc-sensors.vi"("Update Virtual? (T)"=w397, "Caller"=w408, "error in"=w409, "path format (ie. OCS\\\\DB\\\\%s.*)"=w399, "Section (IOnode prefix)"=w398, "IOnodes (AI)"=string[] ["TDRY", "TWET", "UV", "WSPD", "WDIR", "RH"]) -> ("error out"=w404:errorcluster, "results report"=w406:string[])  [unwired: 3 in, 1 out]
          n120 = flat-sequence "LIST INDOOR SECTIONS" {
            tunnel: [w416] -> w403
            frame #0 {
              n121 = call "util-path.vi"("append path (ie. folder\\filename.*)"="ICC" ("dir name")) -> ("error out"=w417:errorcluster, "SelectedPath"=w418:path)  [unwired: 6 in, 3 out]
              n122 = List Folder(path=w418, error in=w417) -> (folder names=w416:string[])  [unwired: 2 in, 3 out]
            }
          }
          n123 = for {
            tunnel: w403 -> [w424] mode=indexing
            tunnel: w404 -> [w431]
            tunnel: [w423] -> w410
            tunnel: [w429] -> w401 mode=concatenating if=w427
            tunnel: w399 -> [w426]
            tunnel: w408 -> [w425]
            tunnel: w397 -> [w422]
            w420 = "_"  # Call I/O from Virtuals
            n124 = Concatenate Strings(w420, w424) -> (w421:string)
            n125 = call "helper-collect-icc-sensors.vi"("Update Virtual? (T)"=w422, "Caller"=w425, "error in"=w431, "path format (ie. OCS\\\\DB\\\\%s.*)"=w426, "Section (IOnode prefix)"=w421, "IOnodes (AI)"=string[] ["TDRY", "TWET", "RH"]) -> ("error out"=w423:errorcluster, "results report"=w429:string[])  [unwired: 3 in, 1 out]
            n126 = Unbundle By Name(w423) -> ("status"=w428:bool)
            n127 = Not(x=w428) -> (.not. x?=w427:bool)
          }
          n128 = Build Array (concatenate)(w406, w401) -> (w402:string[])
          n129 = call "util.DelimitedStringFromArray.vi"("delimiter (Comma)"="," ("delimiter (Tab)"), "params array in"=w402) -> ("delimited string out"=w411:string)  [unwired: 9 in]
        }
        frame "_IO_GET_OUTPUT" {
          w451 = "%s=%d"  # Io, IoValue
          # "\"_IO_GET_STATE\"\nREAD OUTPUT STATE AND SET NUMERIC REGISTER FOR NEXT STATE (COMPARE)"
          n130 = call "variantCtrlStepIoPointer.vi"("procElement"=w444, "error in"=w441, "StepElement in"=w446) -> ("error out"=w435:errorcluster, "I/O Pointer out"=w439:string, "stepElement out"=w445:variant)  [unwired: 5 in, 1 out]
          n131 = call "variantCtrlIo.vi"("menu (Get Param)"=enumVarCtrlIO."IO Get By Key", "error in"=w435, "Key (use IOnode Label if empty )"=w439) -> ("error out"=w437:errorcluster, "IOnode out"=w438:T5)  [unwired: 4 in, 3 out]
          n132 = disable-structure shown="Enabled" {
            disable-tunnel: [w478 w479] -> w447
            disable-tunnel: w445 -> [w477 w479]
            disable-tunnel: w444 -> [w476 _]
            disable-tunnel: [w475 _] -> _
            frame Disabled {
              n133 = call-poly "variantCtrl.polymorphic.vi"("isRequired (T)"=FALSE, "procElement"=w476, "stepElement in"=w477) -> ("File Pointer out"=w475:string, "step\\element out"=w478:variant)  [unwired: 6 in, 1 out]
            }
            frame Enabled {
            }
          }
          n134 = disable-structure shown="Enabled" {
            disable-tunnel: w438 -> [w457 w467]
            disable-tunnel: w437 -> [w455 w468]
            disable-tunnel: [w453 w462] -> w436
            disable-tunnel: [w452 w469] -> w434
            disable-tunnel: w432 -> [_ w461]
            frame Disabled {
              n135 = Unbundle By Name(w457) -> ("Value"=w456:string)
              n136 = case shown="\"ERROR\"" w456 {
                selector: w456 -> [w459 _]
                tunnel: [_ errorcluster {"status"=TRUE, "code"=-1, "source"="OUTPUT IS IN ERROR STATE"} ("error out 2")] -> w454
                tunnel: [w458 _] -> w453
                frame Default {
                  n137 = Decimal String To Number(string=w459) -> (number=w458:i32)  [unwired: 2 in, 1 out]
                }
                frame "ERROR" {
                }
              }
              n138 = Merge Errors(w455, w454) -> (w452:errorcluster)
            }
            frame Enabled {
              n139 = Unbundle By Name(w467) -> ("ADDR"=w465:T6)
              n140 = call "util-address-parser.vi"("ADDR 2"=w465) -> ("Channel"=w464:u8)  [unwired: 9 in, 1 out]
              n141 = Bundle By Name(cluster=T5 {"ADDR"=203, "Label"="Label", "Type"=enum."DI", "Mode"=enum."RIO", "Value"="", "Tags"="", "calibration"=[]} ("IoConf in"), "ADDR"=w465, "Type"=enum.io.type."DI", "Mode"=enum.io.mode."RIO") -> (w470:T5)
              n142 = call "io.interface.serial.vi"("IoConf in"=w470, "Caller"=w461, "error in (no error)"=w468) -> ("DI"=w466:bool[], "error out"=w469:errorcluster)  [unwired: 7 in, 4 out]
              "DI" <- w466
              n143 = Index Array(array=w466, index=w464) -> (element=w463:bool)
              n144 = Boolean To (0,1)(Boolean=w463) -> (0, 1=w462:i16)
            }
          }
          n145 = Format Into String(format string=w451, w439, w436) -> (resulting string=w450:string)  [unwired: 2 in, 1 out]
          n146 = call "variantCtrlNumericRegister.vi"("menu"=enum16{"get", "set"}."set", "error in"=w434, "procNumericRegister in"=w436, "procElement"=w444) -> ("error out"=w442:errorcluster, "procElement out"=w448:variant)  [unwired: 5 in, 1 out]
        }
        frame "_IO_READ" {
          w499 = "%s=%.1f"  # IoPointer, IoValue, IoLogPath
          # "\"_IO_READ\" \nREAD I/O INPUT"
          n147 = call "variantCtrlStepIoPointer.vi"("procElement"=w491, "error in"=w487, "StepElement in"=w493) -> ("error out"=w497:errorcluster, "I/O Pointer out"=w488:string, "stepElement out"=w492:variant)  [unwired: 5 in, 1 out]
          n148 = disable-structure shown="Enabled" {
            disable-tunnel: [w507 w508] -> w500
            disable-tunnel: w497 -> [w506 w508]
            disable-tunnel: [w505 w509] -> w494
            disable-tunnel: w492 -> [w504 w509]
            disable-tunnel: w491 -> [w503 _]
            disable-tunnel: [w502 _] -> w481
            disable-tunnel: FALSE ("isRequired (T)") -> [w501 _]
            frame Enabled {
              n149 = call-poly "variantCtrl.polymorphic.vi"("isRequired (T)"=w501, "procElement"=w503, "error in (no error)"=w506, "stepElement in"=w504) -> ("error out"=w507:errorcluster, "File Pointer out"=w502:string, "step\\element out"=w505:variant)  [unwired: 5 in]
            }
            frame Disabled {
            }
          }
          n150 = call "io.interface.vi"("Caller"=w480, "error in"=w500, "record filename.* (disabled if empty)"=w481, "IO Name in"=w488) -> ("error out"=w483:errorcluster, "Value out"=w485:dbl)  [unwired: 2 in, 4 out]
          n151 = call "proc.util.validateParamExist.vi"("format string"="Missing I/O: %s", "Param Label"=w481) -> ()  [unwired: 9 in, 1 out]
          n152 = Format Into String(format string=w499, w488, w485) -> (resulting string=w498:string)  [unwired: 2 in, 1 out]
          n153 = call "variantCtrlNumericRegister.vi"("menu"=enum16{"get", "set"}."set", "error in"=w483, "procNumericRegister in"=w485, "procElement"=w491) -> ("error out"=w489:errorcluster, "procElement out"=w495:variant)  [unwired: 5 in, 1 out]
        }
        frame "_IO_READ_MANY" {
          n154 = call "variantCtrlStepIoPointer.vi"("procElement"=w522, "error in"=w521, "StepElement in"=w524) -> ("error out"=w526:errorcluster, "I/O Pointer out"=w515:string, "stepElement out"=w523:variant)  [unwired: 5 in, 1 out]
          n155 = call "util.DelimitedStringToArray.vi"("delimiter (,)"=";", "delimitaed string"=w515) -> ("array out"=w517:string[])  [unwired: 9 in]
          n156 = for {
            tunnel: [w530] -> w516 mode=indexing
            shift-right: [w529] -> w519
            shift-left: w526 -> [w531]
            tunnel: w517 -> [w528] mode=indexing
            tunnel: w510 -> [w527]
            n157 = call "io.interface.vi"("Caller"=w527, "error in"=w531, "IO Name in"=w528) -> ("error out"=w529:errorcluster, "Value out"=w530:dbl)  [unwired: 3 in, 4 out]
          }
          n158 = Number To Fractional String(number=w516, precision (6)=i16 2) -> (F-format string=w514:string[])  [unwired: 2 in]
          n159 = call "util.DelimitedStringFromArray.vi"("delimiter (Comma)"=";" ("delimiter (Tab)"), "params array in"=w514) -> ("delimited string out"=w512:string)  [unwired: 9 in]
        }
        frame "_IO_WRITE" {
          w539 = "%s\\\\%s_$date.*"  # prc\\ioname_date.*
          w559 = "%s;%s,%s"  # IoPointer, IoState,recfile
          # "\"_IO_WRITE\"  \nWRITE I/O INPUT"
          n160 = call-poly "variantCtrl.polymorphic.vi"("procElement"=w545, "error in"=w543, "StepElement in"=w554) -> ("error out"=w557:errorcluster, "I/O Pointer out"=w537:string, "stepElement out"=w553:variant)  [unwired: 5 in, 1 out]
          n161 = call "proc.util.enumToStrStepVar.vi"("Step var"=typeStepVarients."stepIoValue" ("proc var")) -> ("String"=w546:string)  [unwired: 10 in]
          n162 = call-poly "variantCtrl.polymorphic.vi"("error in"=w557, "name in"=w546, "Step in"=w553) -> ("error out"=w555:errorcluster, "String Value"=w544:string, "Step out"=w552:variant)  [unwired: 5 in, 1 out]
          n163 = call "util.DO.FromString.vi"("error in"=w555, "initial string"=w544) -> ("error IO"=w550:errorcluster, "output cluster"=w556:cluster{"state":bool, "timeoutSeconds":u16})  [unwired: 8 in]
          n164 = To Variant(anything=w556) -> (Variant=w542:variant)
          n165 = Format Into String(format string=w539, w538, w537) -> (resulting string=w534:string)  [unwired: 2 in, 1 out]
          n166 = call-poly "variantCtrl.polymorphic.vi"("procElement"=w545, "error in (no error)"=w550, "stepElement in"=w552) -> ("error out"=w548:errorcluster, "File Pointer out"=w535:string, "step\\element out"=w551:variant)  [unwired: 6 in]
          n167 = call "step.util.flag-matching.vi"("$string in"=w534) -> ("formated string out"=w533:string)  [unwired: 10 in]
          n168 = Empty String/Path?(string/path=w535) -> (empty?=w536:bool)
          n169 = Select(t=w533, s=w536, f=w535) -> (s? t:f=w532:string)
          n170 = call "io.interface.vi"("Caller"=w538, "error in"=w548, "record filename.* (disabled if empty)"=w532, "IO Value"=w542, "IO Name in"=w537) -> ("error out"=w549:errorcluster)  [unwired: 1 in, 5 out]
          n171 = Format Into String(format string=w559, w537, w544, w532) -> (resulting string=w558:string)  [unwired: 2 in, 1 out]
        }
        frame "_IO_WRITE_BY_REG" {
          w578 = "%s;%d"  # IoPointer, IoState
          # "\"_IO_WRITE\"  \nWRITE I/O INPUT"
          n172 = call-poly "variantCtrl.polymorphic.vi"("procElement"=w568, "error in"=w572, "StepElement in"=w576) -> ("error out"=w563:errorcluster, "I/O Pointer out"=w573:string, "stepElement out"=w575:variant)  [unwired: 5 in, 1 out]
          n173 = call "variantCtrlNumericRegister.vi"("error in"=w563, "procElement"=w568) -> ("error out"=w562:errorcluster, "procNumericRegister out"=w564:dbl, "procElement out"=w569:variant)  [unwired: 7 in]
          n174 = Not Equal To 0?(x=w564) -> (x != 0?=w566:bool)
          n175 = Bundle By Name(cluster=cluster{"state":bool, "timeoutSeconds":u16} {"state"=FALSE, "timeoutSeconds"=0} ("output cluster"), "state"=w566) -> (w565:cluster{"state":bool, "timeoutSeconds":u16})
          n176 = To Variant(anything=w565) -> (Variant=w571:variant)
          n177 = call "io.interface.vi"("Caller"=w561, "error in"=w562, "IO Value"=w571, "IO Name in"=w573) -> ("error out"=w574:errorcluster)  [unwired: 2 in, 5 out]
          n178 = Format Into String(format string=w578, w573, w564) -> (resulting string=w577:string)  [unwired: 2 in, 1 out]
        }
        frame "_IRR_CHECK" {
          # "\"_SUNTIME_CHECK\"  check following special condition and go NEXT if true STAY otherwise"
          n179 = disable-structure shown="Enabled" {
            disable-tunnel: [w599 w603] -> w588
            disable-tunnel: w587 -> [w598 w603]
            disable-tunnel: w582 -> [w597 w602]
            disable-tunnel: [w596 w602] -> w581
            frame Disabled {
              n180 = call "proc.util.enumToStrStepVar.vi"("Step var"=typeStepVarients."stepSeconds" ("proc var")) -> ("String"=w601:string)  [unwired: 10 in]
              n181 = call-poly "variantCtrl.polymorphic.vi"("error in"=w597, "name in"=w601, "variant in"=w598) -> ("error out"=w596:errorcluster, "variant out"=w599:variant)  [unwired: 5 in, 2 out]
            }
            frame Enabled {
            }
          }
          n182 = call "IRR-check-timeframe.vi"("error in"=w581, "Clk"=w594, "ProcName"=w589) -> ("error out"=w580:errorcluster, "ENG.CALL"=w592:cluster{"CMD":T1, "data":variant}, "Report"=w593:string, "Will Irrigate?"=w584:bool)  [unwired: 5 in]
          n183 = Select(t=w592, s=w584, f=w590) -> (s? t:f=w591:cluster{"CMD":T1, "data":variant})
          n184 = Select(t=cluster{"CMD":T2, "data":variant} {"CMD"=enum."NEXT", "data"=variant} ("Next State"), s=w584, f=cluster{"CMD":T2, "data":variant} {"CMD"=enum."STAY", "data"=variant} ("Next State")) -> (s? t:f=w583:cluster{"CMD":T2, "data":variant})
        }
        frame "_JUMP" {
          # "\"_JUMP\"  to another step (pointed by step label)"
          n185 = call-poly "variantCtrl.polymorphic.vi"("procElement (for GET op.)"=w611, "error in"=w605, "stepElement in in"=w613) -> ("error out"=w608:errorcluster, "string out"=w606:string, "stepElement out"=w612:variant)  [unwired: 5 in, 1 out]
          n186 = To Variant(anything=w606) -> (Variant=w607:variant)
          n187 = Bundle By Name(cluster=cluster{"CMD":T2, "data":variant} {"CMD"=enum."JUMP", "data"=variant} ("JUMP"), "data"=w607) -> (w609:cluster{"CMD":T2, "data":variant})
        }
        frame "_COMPLETE" {
          # "\"_JUMP\"  to another step (pointed by step label)"
          n188 = disable-structure shown="Enabled" {
            disable-tunnel: [w626 w627] -> w619
            disable-tunnel: w618 -> [w625 w627]
            disable-tunnel: w617 -> [w624 _]
            disable-tunnel: [w623 _] -> w616
            frame Disabled {
              n189 = call "util-varient-proc-running.vi"("error in"=w624, "Enum"=enum16{"START", "STOP"}."STOP", "Procedure in"=w625) -> ("error out"=w623:errorcluster, "Procedure out"=w626:variant)  [unwired: 7 in]
            }
            frame Enabled {
            }
          }
        }
        frame "_LOG_LAST_REPORT" {
          # "\"_LOG_LAST_REPORT\" save previous report to log file"
          n190 = call-poly "variantCtrl.polymorphic.vi"("procElement"=w649, "error in (no error)"=w648, "stepElement in"=w650) -> ("error out"=w645:errorcluster, "File Pointer out"=w646:string, "step\\element out"=w651:variant)  [unwired: 6 in]
          n191 = call "util-path.vi"("error in"=w645, "Selected Folder (PROCS)"=typePathSelector."DIR_LOG" ("Enum"), "append path (ie. folder\\filename.*)"=w646) -> ("error out"=w629:errorcluster, "SelectedPath"=w636:path, ".extension (.prc)"=w634:string)  [unwired: 4 in, 2 out]
          n192 = call "proc.util.enumToStrProcVar.vi"("Proc var"=typeProcVarientName."procReportPrev" ("proc var")) -> ("String"=w656:string)  [unwired: 10 in]
          n193 = Path To String(path=w636) -> (string=w635:string)
          n194 = call-poly "variantCtrl.polymorphic.vi"("error in"=w645, "name in"=w656, "Step in"=w649) -> ("error out"=w653:errorcluster, "String Value"=w640:string, "Step out"=w654:variant)  [unwired: 5 in, 1 out]
          n195 = Search and Replace String(input string=w635, search string=w634, replace string=".last" ("replace string (\"\")")) -> (result string=w632:string)  [unwired: 5 in, 3 out]
          n196 = Build Array(w640) -> (w637:string[])
          n197 = String To Path(string=w632) -> (path=w631:path)
          n198 = call-poly <vilib>:"Write Delimited Spreadsheet.vi"("file path (dialog if empty)"=w636, "1D data"=w637, "append to file? (new file:F)"=TRUE, "error in (no error)"=w629) -> ("new file path (Not A Path if cancelled)"=w638:path, "error out"=w643:errorcluster)  [unwired: 10 in]
          n199 = call-poly <vilib>:"Write Delimited Spreadsheet.vi"("file path (dialog if empty)"=w631, "1D data"=w637, "error in (no error)"=w629) -> ("error out"=w630:errorcluster)  [unwired: 11 in, 1 out]
          n200 = Merge Errors(w653, w643, w630) -> (w644:errorcluster)
          n201 = Format Into String(format string="(%s),%s", w640, w638) -> (resulting string=w639:string)  [unwired: 2 in, 1 out]
        }
        frame "_LOG_MESSAGE" {
          # "\"_LOG_MESSAGE\" (USER_MSG)\nSave message as a step report. \nCAN BE USED TO MARK A CONDITION IN A PROCEDURE SUCH AS BEGINING/END OR A PROCEDURE"
          n202 = disable-structure shown="Enabled" {
            disable-tunnel: [w694 w714 _] -> w665
            disable-tunnel: [cluster{"CMD":T2, "data":variant} {"CMD"=enum."NEXT", "data"=variant} ("JUMP") cluster{"CMD":T2, "data":variant} {"CMD"=enum."NEXT", "data"=variant} ("JUMP") _] -> w664
            disable-tunnel: w663 -> [w691 w708 _]
            disable-tunnel: w662 -> [w690 w707 _]
            disable-tunnel: [w687 w706 _] -> w661
            disable-tunnel: [w682 w705 _] -> w660
            disable-tunnel: w659 -> [w671 w712 _]
            disable-tunnel: [w667 w710 _] -> w658
            frame Disabled {
              n203 = call-poly "variantCtrl.polymorphic.vi"("procElement"=w671, "error in (no error)"=w690, "stepElement in"=w691) -> ("error out"=w670:errorcluster, "File Pointer out"=w688:string, "step\\element out"=w668:variant)  [unwired: 6 in]
              n204 = call-poly "variantCtrl.polymorphic.vi"("procElement (for GET op.)"=w671, "error in"=w670, "stepElement in in"=w668) -> ("error out"=w669:errorcluster, "string out"=w666:string, "stepElement out"=w667:variant)  [unwired: 5 in, 1 out]
              n205 = disable-structure shown="Enabled" {
                disable-tunnel: [w699 w703] -> w694
                disable-tunnel: [w698 w702] -> w693
                disable-tunnel: [w697 w704] -> w683
                disable-tunnel: w671 -> [w696 w703]
                disable-tunnel: w669 -> [w695 w702]
                disable-tunnel: w666 -> [_ w704]
                frame Disabled {
                  n206 = call "proc.util.enumToStrProcVar.vi"("Proc var"=typeProcVarientName."procReportPrev" ("proc var")) -> ("String"=w701:string)  [unwired: 10 in]
                  n207 = call-poly "variantCtrl.polymorphic.vi"("error in"=w695, "name in"=w701, "Step in"=w696) -> ("error out"=w698:errorcluster, "String Value"=w697:string, "Step out"=w699:variant)  [unwired: 5 in, 1 out]
                }
                frame Enabled {
                }
              }
              n208 = call "util-path.vi"("error in"=w669, "Selected Folder (PROCS)"=typePathSelector."DIR_LOG" ("Enum"), "append path (ie. folder\\filename.*)"=w688) -> ("error out"=w672:errorcluster, "SelectedPath"=w679:path, ".extension (.prc)"=w677:string)  [unwired: 4 in, 2 out]
              n209 = Path To String(path=w679) -> (string=w678:string)
              n210 = Search and Replace String(input string=w678, search string=w677, replace string=".last" ("replace string (\"\")")) -> (result string=w675:string)  [unwired: 5 in, 3 out]
              n211 = String To Path(string=w675) -> (path=w674:path)
              n212 = Build Array(w683) -> (w680:string[])
              n213 = call-poly <vilib>:"Write Delimited Spreadsheet.vi"("file path (dialog if empty)"=w674, "1D data"=w680, "error in (no error)"=w672) -> ("error out"=w673:errorcluster)  [unwired: 11 in, 1 out]
              n214 = call-poly <vilib>:"Write Delimited Spreadsheet.vi"("file path (dialog if empty)"=w679, "1D data"=w680, "append to file? (new file:F)"=TRUE, "error in (no error)"=w672) -> ("new file path (Not A Path if cancelled)"=w681:path, "error out"=w686:errorcluster)  [unwired: 10 in]
              n215 = Merge Errors(w693, w686, w673) -> (w687:errorcluster)
              n216 = Format Into String(format string="(%s),%s", w683, w681) -> (resulting string=w682:string)  [unwired: 2 in, 1 out]
            }
            frame Enabled {
              n217 = call-poly "variantCtrl.polymorphic.vi"("procElement (for GET op.)"=w712, "error in"=w707, "stepElement in in"=w708) -> ("error out"=w711:errorcluster, "string out"=w709:string, "stepElement out"=w710:variant)  [unwired: 5 in, 1 out]
              n218 = disable-structure shown="Enabled" {
                disable-tunnel: [w719 w723] -> w714
                disable-tunnel: [w718 w722] -> w706
                disable-tunnel: [w717 w724] -> w705
                disable-tunnel: w712 -> [w716 w723]
                disable-tunnel: w711 -> [w715 w722]
                disable-tunnel: w709 -> [_ w724]
                frame Disabled {
                  n219 = call "proc.util.enumToStrProcVar.vi"("Proc var"=typeProcVarientName."procReportPrev" ("proc var")) -> ("String"=w721:string)  [unwired: 10 in]
                  n220 = call-poly "variantCtrl.polymorphic.vi"("error in"=w715, "name in"=w721, "Step in"=w716) -> ("error out"=w718:errorcluster, "String Value"=w717:string, "Step out"=w719:variant)  [unwired: 5 in, 1 out]
                }
                frame Enabled {
                }
              }
            }
            frame Disabled {
            }
          }
        }
        frame "_REC_DELETE", "_REC_MOVE" {
          w737 = typePathSelector."DIR_RECORD" ("Selected Folder (PROCEDURE_DIR)")
          w743 = "%s"  # Files, Operation
          # "\"_RECORD_FILE_DELETE\", \"_RECORD_FILE_MOVE\" (SRC,DEST)"
          n221 = call-poly "variantCtrl.polymorphic.vi"("isRequired (T)"=FALSE, "procElement"=w745, "error in (no error)"=w744, "stepElement in"=w746) -> ("error out"=w730:errorcluster, "File Pointer out"=w727:string, "step\\element out"=w747:variant)  [unwired: 5 in]
          n222 = call "util.DelimitedStringToArray.vi"("delimitaed string"=w727) -> ("array out"=w739:string[])  [unwired: 10 in]
          n223 = Format Into String(format string=w743, w727) -> (resulting string=w742:string)  [unwired: 2 in, 1 out]
          n224 = Index Array(array=w739) -> (element #1=w736:string, element #2=w738:string)  [unwired: 2 in]
          n225 = call "util-path.vi"("error in"=w730, "Selected Folder (PROCS)"=w737, "append path (ie. folder\\filename.*)"=w736) -> ("error out"=w735:errorcluster, "SelectedPath"=w733:path)  [unwired: 4 in, 3 out]
          n226 = call "util-path.vi"("Create Folders?(F)"=TRUE, "error in"=w730, "Selected Folder (PROCS)"=w737, "append path (ie. folder\\filename.*)"=w738) -> ("error out"=w734:errorcluster, "SelectedPath"=w732:path)  [unwired: 3 in, 3 out]
          n227 = Merge Errors(w735, w734) -> (w731:errorcluster)
          n228 = case shown="\"_REC_MOVE\"" w728 {
            tunnel: w733 -> [_ w754 w759 w762]
            tunnel: w732 -> [_ w753 w758 _]
            tunnel: w731 -> [w749 w752 w757 w761]
            tunnel: [w749 w751 w756 w760] -> w729
            frame "__NO-OP", Default {
            }
            frame "_REC_MOVE" {
              n229 = Move(source path=w754, error in=w752, 9:FALSE ("overwrite (F)"), 10:w753) -> (error out=w751:errorcluster)  [unwired: 1 in, 2 out]
            }
            frame "_REC_COPY" {
              n230 = Copy(8:w757, 9:FALSE ("overwrite (F)"), 10:w758, 11:w759) -> (0:w756:errorcluster)  [unwired: 1 in, 2 out]
            }
            frame "_REC_DELETE" {
              n231 = Delete(path (use dialog)=w762, error in=w761) -> (error out=w760:errorcluster)  [unwired: 3 in, 2 out]
            }
          }
          n232 = Merge Errors(w729) -> (w741:errorcluster)
        }
        frame "_SCHEDULE" {
          # "\"_SCHEDULE\" \nInput: encoded string of cluster of sched-mode and sched-pairs array"
          n233 = call "sched-check.vi"("error in"=w766, "stepElement in"=w769, "clk"=w764) -> ("error out"=w768:errorcluster, "stepElement out"=w771:variant, "resulting string"=w767:string, "Next State"=w770:cluster{"CMD":T2, "data":variant})  [unwired: 5 in]
        }
        frame "_SCHEDULE_DAILY" {
          w775 = "%s"  # IoPointer, IoState
          # "\"_SCHED_DAILY\" CHECK IF CLOCK IS IN SCHEDULED TIME BEFORE CONTINUE TO NEXT STEP\n\nSTEP ARGS:"
          n234 = call "proc.util.enumToStrProcVar.vi"("Proc var"=typeProcVarientName."procNameID" ("proc var")) -> ("String"=w792:string)  [unwired: 10 in]
          n235 = call-poly "variantCtrl.polymorphic.vi"("error in"=w791, "name in"=w792, "Step in"=w794) -> ("error out"=w786:errorcluster, "String Value"=w779:string, "Step out"=w795:variant)  [unwired: 5 in, 1 out]
          n236 = Bundle By Name(cluster=cluster{"CMD":T1, "data":variant} {"CMD"=enum."ENG.PROC.STOP", "data"=variant} ("element"), "data"=w779) -> (w796:cluster{"CMD":T1, "data":variant})
          n237 = call "proc.util.enumToStrStepVar.vi"("Step var"=typeStepVarients."stepTimeString") -> ("String"=w790:string)  [unwired: 10 in]
          n238 = call-poly "variantCtrl.polymorphic.vi"("error in"=w786, "name in"=w790, "Step in"=w787) -> ("error out"=w777:errorcluster, "String Value"=w773:string, "Step out"=w788:variant)  [unwired: 5 in, 1 out]
          n239 = call "util-timestring-to-timestamp.vi"("error in"=w777, "String Value"=w773) -> ("error out"=w776:errorcluster, "Time Stamp"=w778:timestamp)  [unwired: 8 in]
          n240 = Bundle By Name(cluster=T12 {"Proc Name"="", "value"={"Enable"=TRUE, "Time"=timestamp(0 s since 1904-01-01)}}, "Proc Name"=w779, "value.Time"=w778, "value.Enable"=TRUE) -> (w780:T12)
          n241 = Bundle By Name(cluster=cluster{"data":variant, "Enum":T13} {"data"=variant, "Enum"=enum."SCHED.REGISTER"} ("element"), "data"=w780) -> (w782:cluster{"data":variant, "Enum":T13})
          n242 = global read "globals-engine.vi" "Q-Sched"() -> (w784:refnum<queue>)
          n243 = Enqueue Element(queue=w784, element=w782, error in (no error)=w776) -> (error out=w785:errorcluster)  [unwired: 1 in, 2 out]
          n244 = Format Into String(format string=w775, w773) -> (resulting string=w774:string)  [unwired: 2 in, 1 out]
        }
        frame "CLK_COMPARE" {
          # "TO BE DEFINED - SHOULD PROVIDE TIME COMPARISON ???"
          n245 = call "proc.util.compare.vi"("error in"=w801, "stepElement in"=w802, "Input"=w803, "procElement in"=w806) -> ("error out"=w800:errorcluster, "stepElement out"=w805:variant, "resulting string"=w799:string, "procElement out"=w807:variant, "Next State"=w804:cluster{"CMD":T2, "data":variant})  [unwired: 3 in]
        }
        frame "PROC_COMPLETION_CHECK" {
          w816 = cluster{"CMD":T2, "data":variant} {"CMD"=enum."NEXT", "data"=variant}  # NEXT
          w808 = cluster{"CMD":T2, "data":variant} {"CMD"=enum."PREV", "data"=variant}  # PREV
          # "\"PROC_RUN_IF_OFF\"  NEXT if procIsRunning==OFF and JUMP otherwise"
          n246 = disable-structure shown="Disabled" {
            disable-tunnel: w826 -> [w833 _]
            disable-tunnel: [w832 _] -> w825
            disable-tunnel: [w828 _] -> w818
            disable-tunnel: w815 -> [w827 _]
            frame Disabled {
              # "needed only if need to check"
              n247 = call "proc.util.enumToStrStepVar.vi"("Step var"=typeStepVarients."stepProcPointer") -> ("String"=w831:string)  [unwired: 10 in]
              n248 = call-poly "variantCtrl.polymorphic.vi"("error in"=w827, "name in"=w831, "Step in"=w833) -> ("error out"=w828:errorcluster, "String Value"=w829:string, "Step out"=w832:variant)  [unwired: 5 in, 1 out]
              n249 = To Variant(anything=w829) -> ()  [unwired: 1 out]
            }
            frame Enabled {
            }
          }
          n250 = call "proc.util.enumToStrProcVar.vi"("Proc var"=typeProcVarientName."procRegisterString" ("proc var")) -> ("String"=w824:string)  [unwired: 10 in]
          n251 = call-poly "variantCtrl.polymorphic.vi"("error in"=w815, "name in"=w824, "Step in"=w821) -> ("error out"=w820:errorcluster, "String Value"=w813:string, "Step out"=w822:variant)  [unwired: 5 in, 1 out]
          n252 = Match Pattern(string=w813, regular expression="=") -> (after substring=w812:string)  [unwired: 1 in, 3 out]
          n253 = Equal?(x=w812, y="OFF") -> (x = y?=w810:bool)
          n254 = Select(t=w816, s=w810, f=w808) -> (s? t:f=w819:cluster{"CMD":T2, "data":variant})
          n255 = Merge Errors(w820, w818) -> (w817:errorcluster)
        }
        frame "PROC_COMPLETION_LOAD" {
          # "eng call should update this field with the proc status ON/OFF"
          # "PROC_COMPLETION_LOAD\nmake engine call to check if procLabel\n \"PROC_WAIT\"  send PROC-WAIT cmd to QController. \nNext state should check string Register for status: \"procLabel=ON/OFF\""
          n256 = call "proc.util.enumToStrStepVar.vi"("Step var"=typeStepVarients."stepProcPointer") -> ("String"=w858:string)  [unwired: 10 in]
          n257 = call "proc.util.enumToStrProcVar.vi"("Proc var"=typeProcVarientName."procNameID" ("proc var")) -> ("String"=w855:string)  [unwired: 10 in]
          n258 = call-poly "variantCtrl.polymorphic.vi"("error in"=w850, "name in"=w855, "Step in"=w853) -> ("error out"=w849:errorcluster, "String Value"=w843:string, "Step out"=w841:variant)  [unwired: 5 in, 1 out]
          n259 = call-poly "variantCtrl.polymorphic.vi"("error in"=w850, "name in"=w858, "Step in"=w860) -> ("error out"=w856:errorcluster, "String Value"=w842:string, "Step out"=w859:variant)  [unwired: 5 in, 1 out]
          n260 = Format Into String(format string="%s", w842) -> (resulting string=w851:string)  [unwired: 2 in, 1 out]
          n261 = Merge Errors(w849, w856) -> (w839:errorcluster)
          n262 = Bundle By Name(cluster=T14 {"callerProc"="", "procPointer"=""}, "callerProc"=w843, "procPointer"=w842) -> (w844:T14)
          n263 = call "proc.util.enumToStrProcVar.vi"("Proc var"=typeProcVarientName."procRegisterString" ("proc var")) -> ("String"=w837:string)  [unwired: 10 in]
          n264 = Bundle By Name(cluster=cluster{"CMD":T1, "data":variant} {"CMD"=enum."ENG.PROC.ISRUNNING", "data"=variant} ("element"), "data"=w844) -> (w848:cluster{"CMD":T1, "data":variant})
          n265 = call-poly "variantCtrl.polymorphic.vi"("menu in (get)"=enum16{"get", "set"}."set", "error in"=w839, "String Value"="", "name in"=w837, "Step in"=w841) -> ("error out"=w838:errorcluster, "Step out"=w840:variant)  [unwired: 3 in, 2 out]
        }
        frame "PROC_START".."PROC_LOAD" {
          # "\"PROC_START\", \"PROC_STOP\", \"PROC_LOAD\"  \nsend engine call to start/stop/load procedure"
          n266 = case shown="\"PROC_STOP\"" w864 {
            tunnel: [cluster{"CMD":T1, "data":variant} {"CMD"=enum."ENG.NO-OP", "data"=variant} ("element") cluster{"CMD":T1, "data":variant} {"CMD"=enum."ENG.PROC.START", "data"=variant} ("element") cluster{"CMD":T1, "data":variant} {"CMD"=enum."ENG.PROC.STOP", "data"=variant} ("element") cluster{"CMD":T1, "data":variant} {"CMD"=enum."ENG.PROC.RELOAD-BY-NAME", "data"=variant} ("element")] -> w863
            frame Default {
            }
            frame "PROC_START" {
            }
            frame "PROC_STOP" {
            }
            frame "PROC_LOAD" {
            }
          }
          n267 = call-poly "variantCtrl.polymorphic.vi"("procElement (for GET op.)"=w862, "error in"=w867, "stepElement in in"=w870) -> ("error out"=w868:errorcluster, "string out"=w861:string, "stepElement out"=w869:variant)  [unwired: 5 in, 1 out]
          n268 = Bundle By Name(cluster=w863, "data"=w861) -> (w865:cluster{"CMD":T1, "data":variant})
        }
        frame "UNIT_CHECK" {
          # "\"NUTRITION_CHECK\" (UNIT_INDEX)\nstart wash in and prepare for wash out and close"
          n269 = disable-structure shown="Enabled" {
            disable-tunnel: [w902 w903] -> w893
            disable-tunnel: w892 -> [w901 w903]
            disable-tunnel: w882 -> [w900 _]
            disable-tunnel: [w899 _] -> w880
            frame Disabled {
              n270 = call-poly "enumToStr.vi"("Step var"=typeStepVarients."stepUnitIndex") -> ("String"=w898:string)  [unwired: 10 in]
              n271 = call-poly "variantCtrl.polymorphic.vi"("error in"=w900, "name in"=w898, "variant in"=w901) -> ("error out"=w899:errorcluster, "variant out"=w902:variant)  [unwired: 5 in, 2 out]
            }
            frame Enabled {
            }
          }
          n272 = call "flow-builder-nutrition-check.vi"("clk"=w879) -> ("error out"=w883:errorcluster, "Check Report"=w878:string, "intructions out"=w877:variant[])  [unwired: 8 in]
          n273 = Array Size(array=w877) -> (size(s)=w876:i32)
          n274 = Bundle By Name(cluster=T15 {"ProcName"="", "instructions"=[]}, "ProcName"=w887, "instructions"=w877) -> (w886:T15)
          n275 = Greater Than 0?(x=w876) -> (x > 0?=w875:bool)
          n276 = Bundle By Name(cluster=cluster{"CMD":T1, "data":variant} {"CMD"=enum."ENG.PROC.INSERT-STEPS", "data"=variant} ("element"), "data"=w886) -> (w890:cluster{"CMD":T1, "data":variant})
          n277 = Select(t=w890, s=w875, f=w891) -> (s? t:f=w889:cluster{"CMD":T1, "data":variant})
          n278 = Merge Errors(w880, w883) -> (w881:errorcluster)
          n279 = Format Into String(format string="Unit check: %s", w878) -> (resulting string=w884:string)  [unwired: 2 in, 1 out]
        }
        frame "UNIT_DOSE" {
          # "\"NUTRITION_DOSE\" (unitIndex, output, dosingTime)\nverify daily dosing limit and start doser if not reached limit. every dosing is registered and accumulated in a daily file"
          n280 = stacked-sequence {
            seq-local: [w917 _] -> [_ w938]
            seq-local: [w916 _] -> [_ w942]
            tunnel: [_ cluster{"CMD":T2, "data":variant} {"CMD"=enum."NEXT", "data"=variant} ("Next State")] -> w913
            tunnel: [w915 _] -> w912
            tunnel: w911 -> [w928 _]
            tunnel: w910 -> [_ w951]
            tunnel: [_ w949] -> w909
            tunnel: w908 -> [_ w939]
            tunnel: [w918 _] -> w907
            tunnel: [_ w937] -> w905
            tunnel: [_ w943] -> w904
            frame #0 {
              # "make sure not pass the daily limiter.\nif final dose is above daily limit then \ninject only the difference to make it \nto the dily limit"
              # "validate daily limit"
              n281 = call-poly "enumToStr.vi"("Step var"=typeStepVarients."stepUnitIndex") -> ("String"=w927:string)  [unwired: 10 in]
              n282 = call-poly "variantCtrl.polymorphic.vi"("name in"=w927, "variant in"=w928) -> ("error out"=w922:errorcluster, "number"=w925:dbl, "variant out"=w923:variant)  [unwired: 6 in, 1 out]
              n283 = To Long Integer(number=w925) -> (32bit integer=w917:i32)
              n284 = call-poly "enumToStr.vi"("Step var"=typeStepVarients."stepIoPointer") -> ("String"=w924:string)  [unwired: 10 in]
              n285 = call-poly "variantCtrl.polymorphic.vi"("error in"=w922, "name in"=w924, "Step in"=w923) -> ("error out"=w919:errorcluster, "String Value"=w916:string, "Step out"=w920:variant)  [unwired: 5 in, 1 out]
              n286 = disable-structure shown="Enabled" {
                disable-tunnel: w920 -> [w931 w935]
                disable-tunnel: w919 -> [w930 w934]
                disable-tunnel: [w929 w934] -> w918
                disable-tunnel: [_ w935] -> w915
                frame Disabled {
                  n287 = call-poly "enumToStr.vi"("Step var"=typeStepVarients."stepSeconds") -> ("String"=w932:string)  [unwired: 10 in]
                  n288 = call-poly "variantCtrl.polymorphic.vi"("error in"=w930, "name in"=w932, "variant in"=w931) -> ("error out"=w929:errorcluster)  [unwired: 5 in, 3 out]
                }
                frame Enabled {
                }
              }
            }
            frame #1 {
              n289 = Build Array(w942) -> (w946:string[])
              n290 = call "helper-unit-dose.vi"("output"=w942, "Unit Index"=w938, "Proc Name"=w939) -> ("error out"=w944:errorcluster, "resulting string"=w943:string, "Actual Dose in Seconds"=w941:i32)  [unwired: 6 in]
              n291 = Greater Than 0?(x=w941) -> (x > 0?=w945:bool)
              n292 = call "flow-builder-nutrition-dose.vi"("Proc Name (empty: bypass logging)"=w939, "Unit Index"=w938, "Digital Timeout"=w941, "OUTPUT(+AUX)"=w946) -> ("error out"=w936:errorcluster, "intructions out"=w940:variant[])  [unwired: 6 in]
              n293 = Bundle By Name(cluster=T15 {"ProcName"="", "instructions"=[]}, "ProcName"=w939, "instructions"=w940) -> (w947:T15)
              n294 = Merge Errors(w936, w944) -> (w937:errorcluster)
              n295 = Bundle By Name(cluster=cluster{"CMD":T1, "data":variant} {"CMD"=enum."ENG.PROC.INSERT-STEPS", "data"=variant} ("element"), "data"=w947) -> (w950:cluster{"CMD":T1, "data":variant})
              n296 = Select(t=w950, s=w945, f=w951) -> (s? t:f=w949:cluster{"CMD":T1, "data":variant})
            }
          }
          n297 = Merge Errors(w907, w905) -> (w906:errorcluster)
        }
        frame "UNIT_SAMPLE" {
          # "\"UNIT_SAMPLE\"  (UNIT_INDEX)\n read sensors and add unit dose steps"
          n298 = call-poly "enumToStr.vi"("Step var"=typeStepVarients."stepUnitIndex") -> ("String"=w967:string)  [unwired: 10 in]
          n299 = call-poly "variantCtrl.polymorphic.vi"("name in"=w967, "variant in"=w968) -> ("number"=w959:dbl, "variant out"=w969:variant)  [unwired: 6 in, 2 out]
          n300 = To Long Integer(number=w959) -> (32bit integer=w962:i32)
          n301 = call "flow-builder.nutrition-sample.vi"("Proc Name"=w956, "Unit Index"=w962) -> ("error out"=w958:errorcluster, "status"=w957:string, "intructions out"=w955:variant[])  [unwired: 5 in, 2 out]
          n302 = Bundle By Name(cluster=T15 {"ProcName"="", "instructions"=[]}, "ProcName"=w956, "instructions"=w955) -> (w960:T15)
          n303 = Bundle By Name(cluster=cluster{"CMD":T1, "data":variant} {"CMD"=enum."ENG.PROC.INSERT-STEPS", "data"=variant} ("element"), "data"=w960) -> (w964:cluster{"CMD":T1, "data":variant})
          n304 = Select(t=w964, s=TRUE, f=w965) -> (s? t:f=w963:cluster{"CMD":T1, "data":variant})
        }
      }
      n305 = call "proc.util.errorDescriptor.vi"("stepElement"=w30, "procElement"=w31, "NextState in"=w34, "error in"=w20) -> ("nextState out"=w33:cluster{"CMD":T2, "data":variant}, "error out"=w32:errorcluster)  [unwired: 5 in, 1 out]
      n306 = call "proc.util.enumToStrProcVar.vi"("Proc var"=typeProcVarientName."procReport" ("proc var")) -> ("String"=w28:string)  [unwired: 10 in]
      n307 = Select(t=FALSE, s=w20, f=w18) -> (s? t:f=w17:bool)
      n308 = call-poly "variantCtrl.polymorphic.vi"("menu in (get)"=enum16{"get", "set"}."set", "String Value"=w22, "name in"=w28, "Step in"=w31) -> ("Step out"=w47:variant)  [unwired: 4 in, 3 out]
      n309 = Build Array(w47, w30) -> (w46:variant[])
    }
  }
  "error out" <- w12
  "Next State in" <- w13
  "ENG.CALL" <- w5
  "continue?" <- w1
  n310 = flat-sequence {
    frame #0 {
      (unwired) typeProcVarientName."procModule" ("proc var")
      (unwired) typeProcVarientName."procModuleID" ("proc var")
    }
  }
  n311 = Bundle(w11) -> (→"HeaderElement out":cluster{variant[]})  [unwired: 1 in]
